vi "Camera.vi"(5 "Camera Notifiers":T2, 6 "Auto Settings?":bool, 7 "Refnums":T4, 8 "Error In":errorcluster, 9 "Set Camera ID":u32, 10 "Settings":T5={"Pixel clock"=20, "Frame rate"=30.0, "Exposure time"=33.21525, "Master Gain"=0, "Red Gain"=0, "Green Gain"=0, "Blue Gain"=0, "Auto Gain"=FALSE, "White-balance"=FALSE, "Color Correction"=FALSE} {"Blue Gain" min=0 max=100 step=1 scale=0.0..100.0; "Green Gain" min=0 max=100 step=1 scale=0.0..100.0; "Red Gain" min=0 max=100 step=1 scale=0.0..100.0; "Master Gain" min=0 max=100 step=1 scale=0.0..100.0; "Exposure time" min=0.271 max=424.65700000000004 step=0.271 scale=0.271..424.65700000000004 scale format="%#.3g"; "Frame rate" min=2.3503419747573275 max=2.3503419747573275 step=0.000271 scale=2.3503419747573275..2.5853761722330604 scale format="%^#_3g"; "Pixel clock" min=5 max=43 step=1 scale=5.0..43.0}, 11 "Function":T7=enum."Update Settings") -> (0 "Error Out":errorcluster, 2 "Image":T3(plugin-control), 3 "Image":T6)   [LabVIEW 2014]
uses:
  Camera Functions.ctl
  Camera Img Data.ctl
  Camera Settings.ctl
  Camera Refnums.ctl
  support/Instrument Status.ctl
  Camera Notifiers.ctl
  support/Instrument Status State.ctl
  <vilib>/vision/NI_Vision_Development_Module.lvlib
panel:
  out "Instrument Status":T1
  out "Camera Handle":u32=1
  # "LICENSED MATERIALS – PROPERTY OF IBM\nCopyright IBM Corp. 2016,\nALL RIGHTS RESERVED"
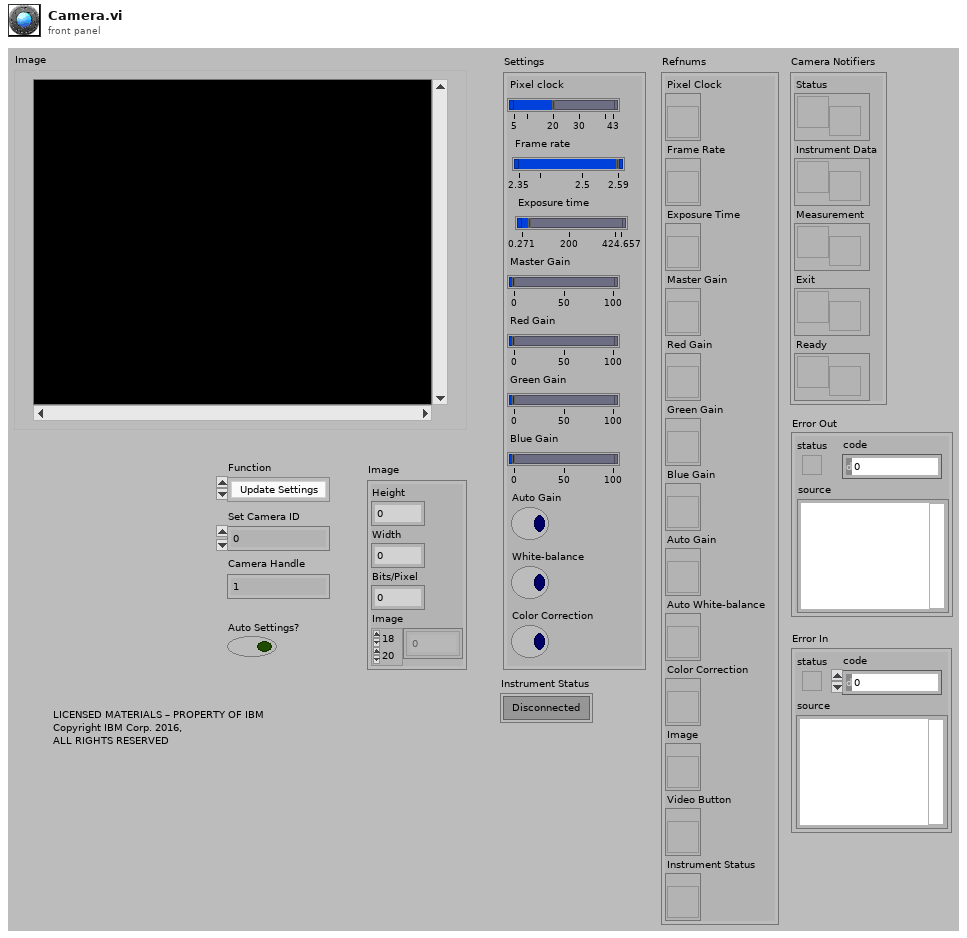
[diagram p1: front panel]
types:
  T1 = typedef "Instrument Status.ctl" = bool
  T2 = typedef "Camera Notifiers.ctl" = cluster{"Status":refnum<notifier>, "Instrument Data":refnum<notifier>, "Measurement":refnum<notifier>, "Exit":refnum<notifier>, "Ready":refnum<notifier>}
  T3 = typedef "IMAQ Image.ctl" = refnum<image>
  T4 = typedef "Camera Refnums.ctl" = cluster{"Pixel Clock":refnum<vi>, "Frame Rate":refnum<vi>, "Exposure Time":refnum<vi>, "Master Gain":refnum<vi>, "Red Gain":refnum<vi>, "Green Gain":refnum<vi>, "Blue Gain":refnum<vi>, "Auto Gain":refnum<vi>, "Auto White-balance":refnum<vi>, "Color Correction":refnum<vi>, "Image":refnum<vi>, "Video Button":refnum<vi>, "Instrument Status":refnum<vi>}
  T5 = typedef "Camera Settings.ctl" = cluster{"Pixel clock":i32, "Frame rate":dbl, "Exposure time":dbl, "Master Gain":i32, "Red Gain":i32, "Green Gain":i32, "Blue Gain":i32, "Auto Gain":bool, "White-balance":bool, "Color Correction":bool}
  T6 = typedef "Camera Img Data.ctl" = cluster{"Height":i32, "Width":i32, "Bits/Pixel":i32, "Image":u32[][]}
  T7 = typedef "Camera Functions.ctl" = enum16{"Connect", "Start Live", "Acquire", "Update Settings", "Update Settings2", "Stop Live", "Disconnect", "Update Refnums"}
  T8 = enum16{"All", "Limits", "Value", "User Enablement"}
  T9 = typedef "Instrument Status State.ctl" = enum16{"Unknown", "Idle", "Standby", "Configuring", "Measuring", "Moving", "Disconnected"}
  T10 = typedef "Image Type" = u32
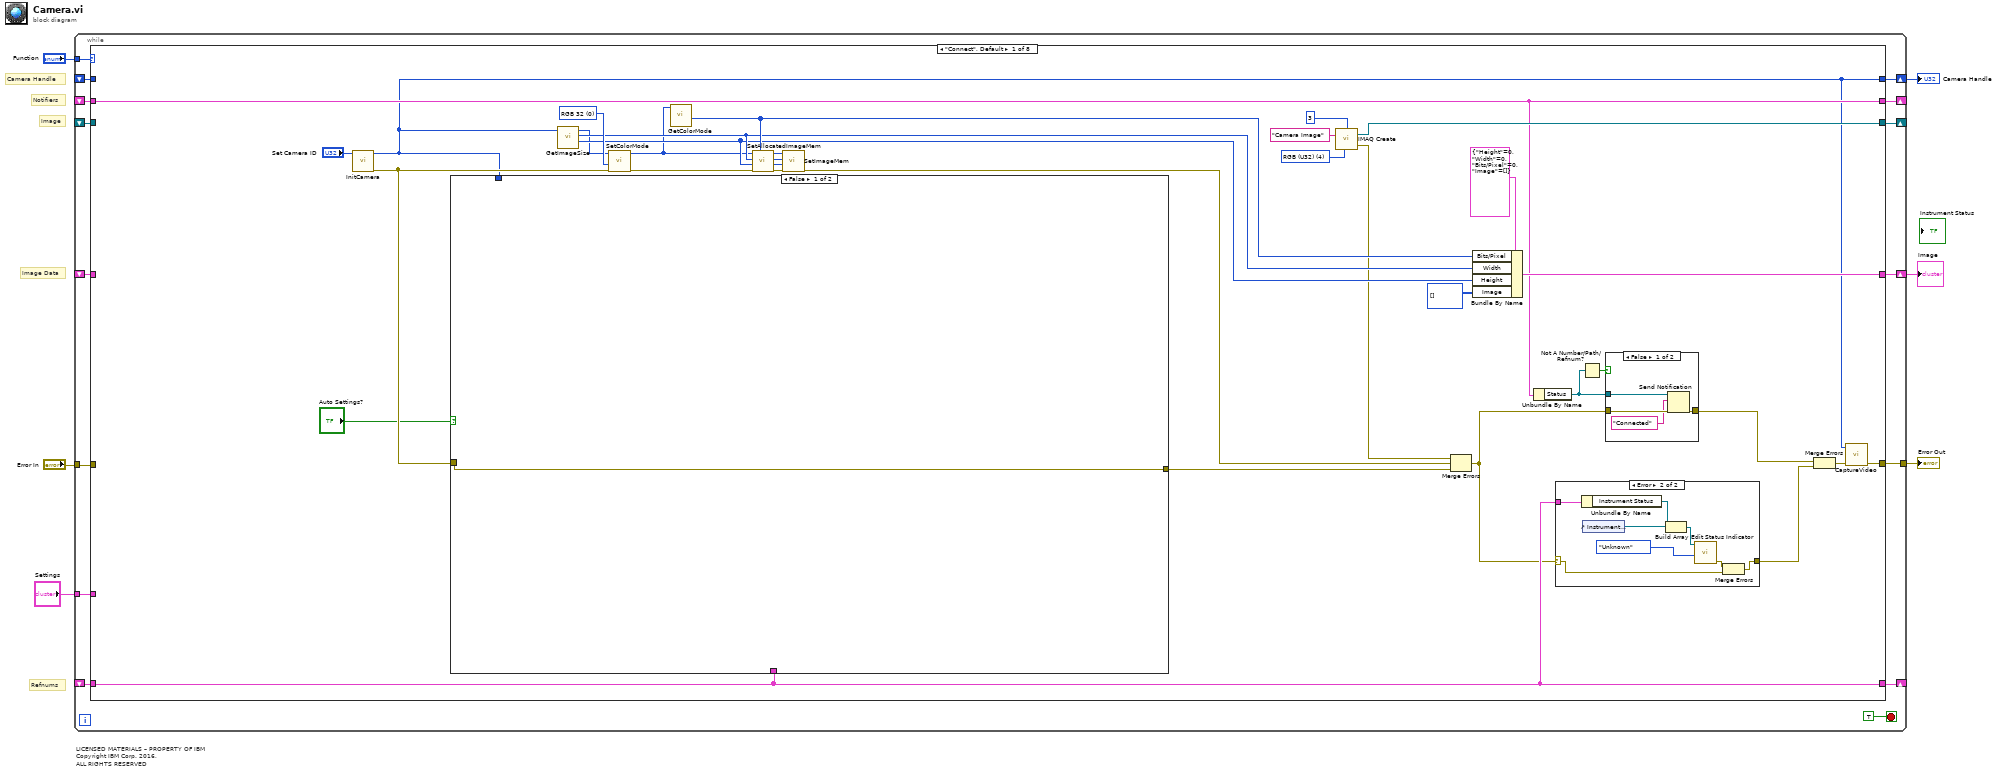
[diagram p0: block diagram]
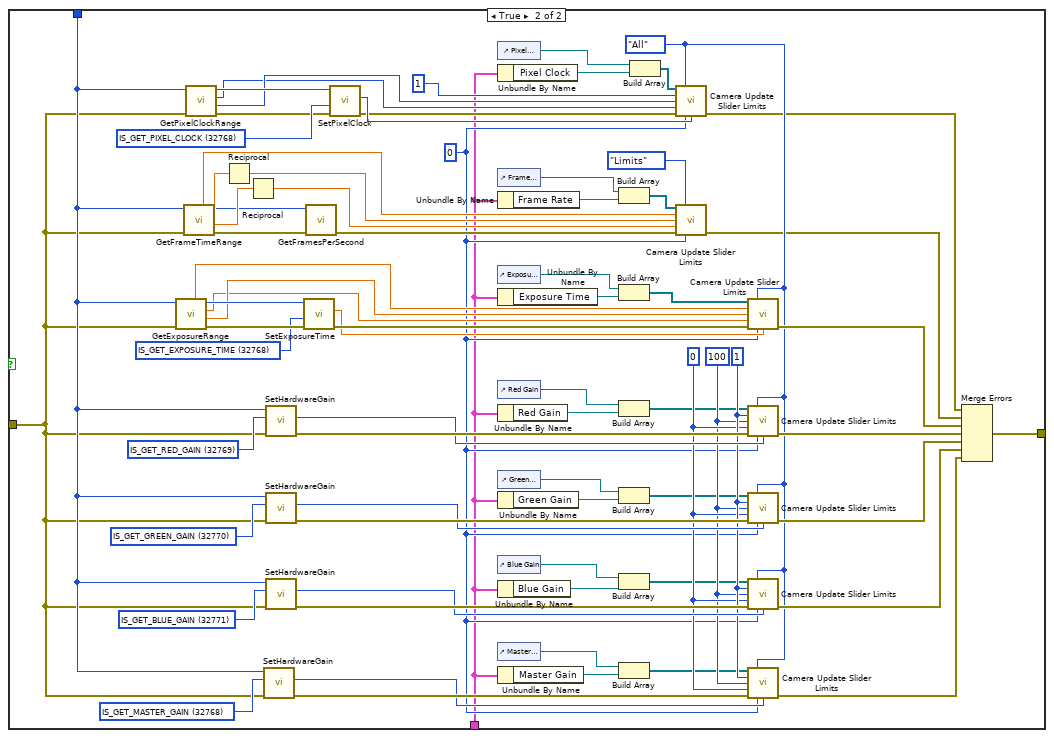
[diagram p2: hidden frame]
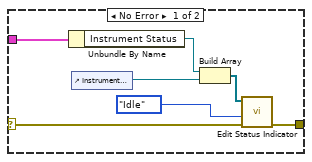
[diagram p3: hidden frame]
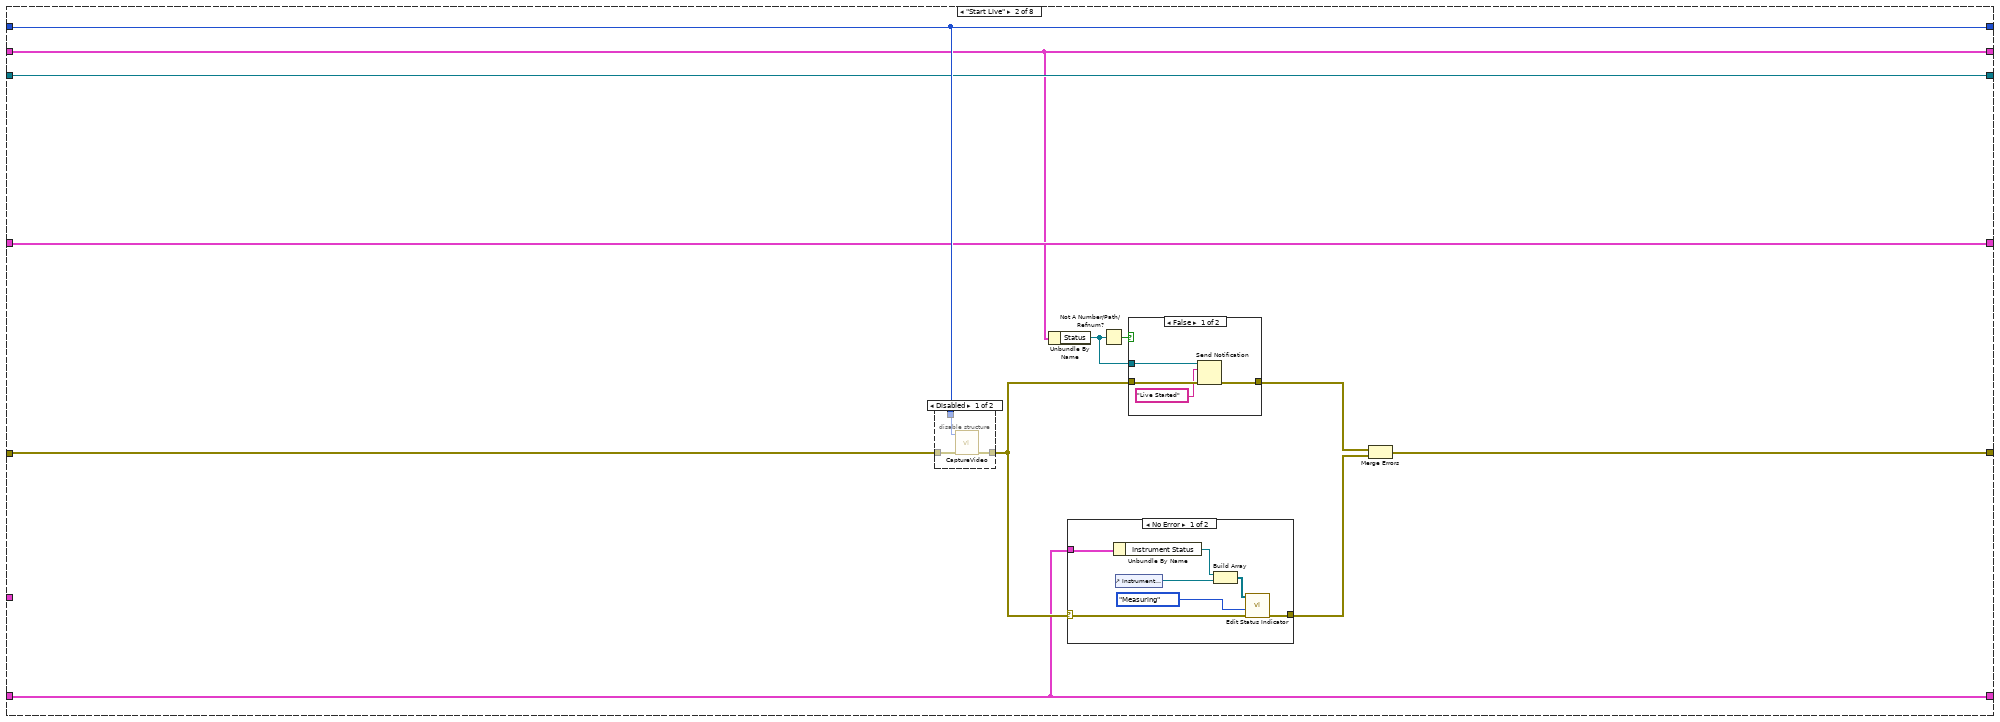
[diagram p5: hidden frame]
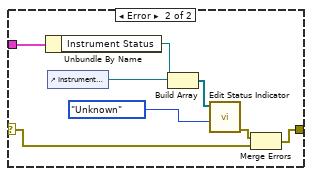
[diagram p7: hidden frame]
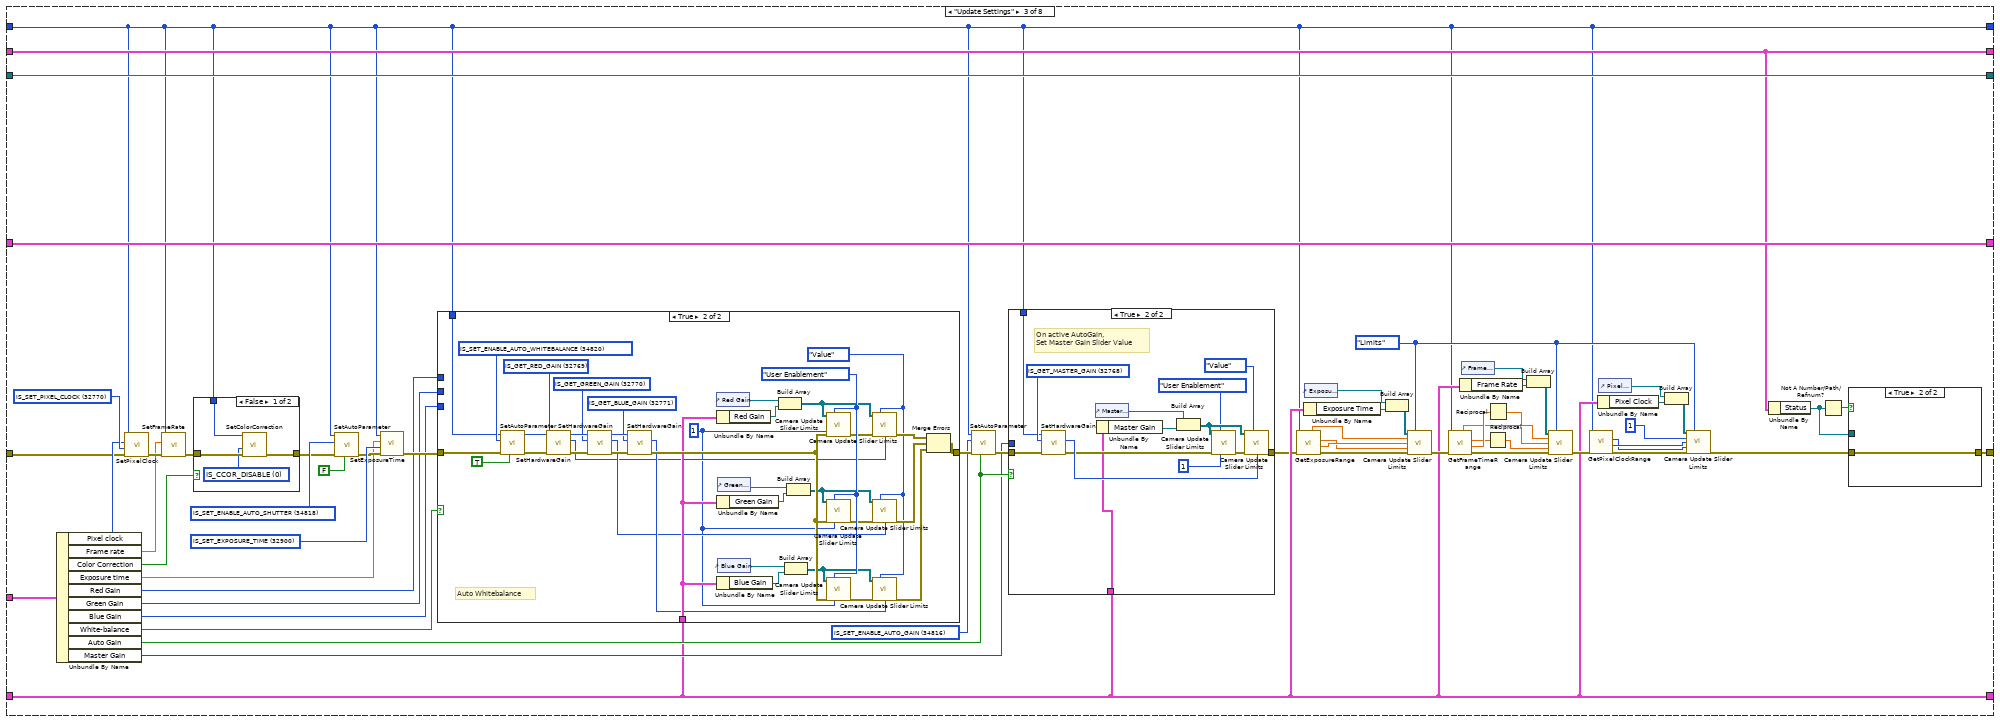
[diagram p9: hidden frame]
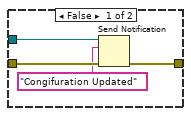
[diagram p10: hidden frame]
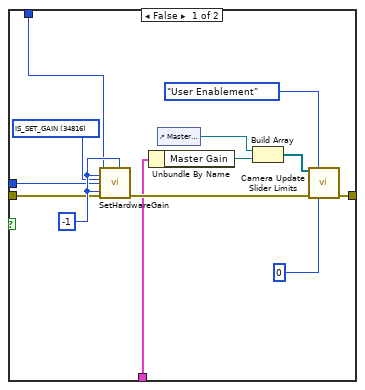
[diagram p11: hidden frame]
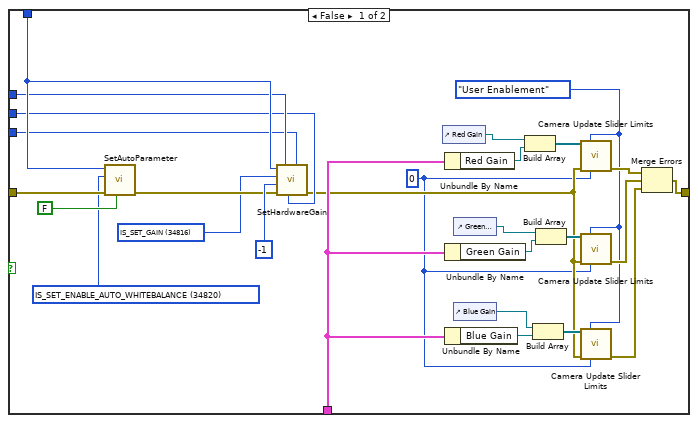
[diagram p12: hidden frame]
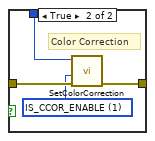
[diagram p13: hidden frame]
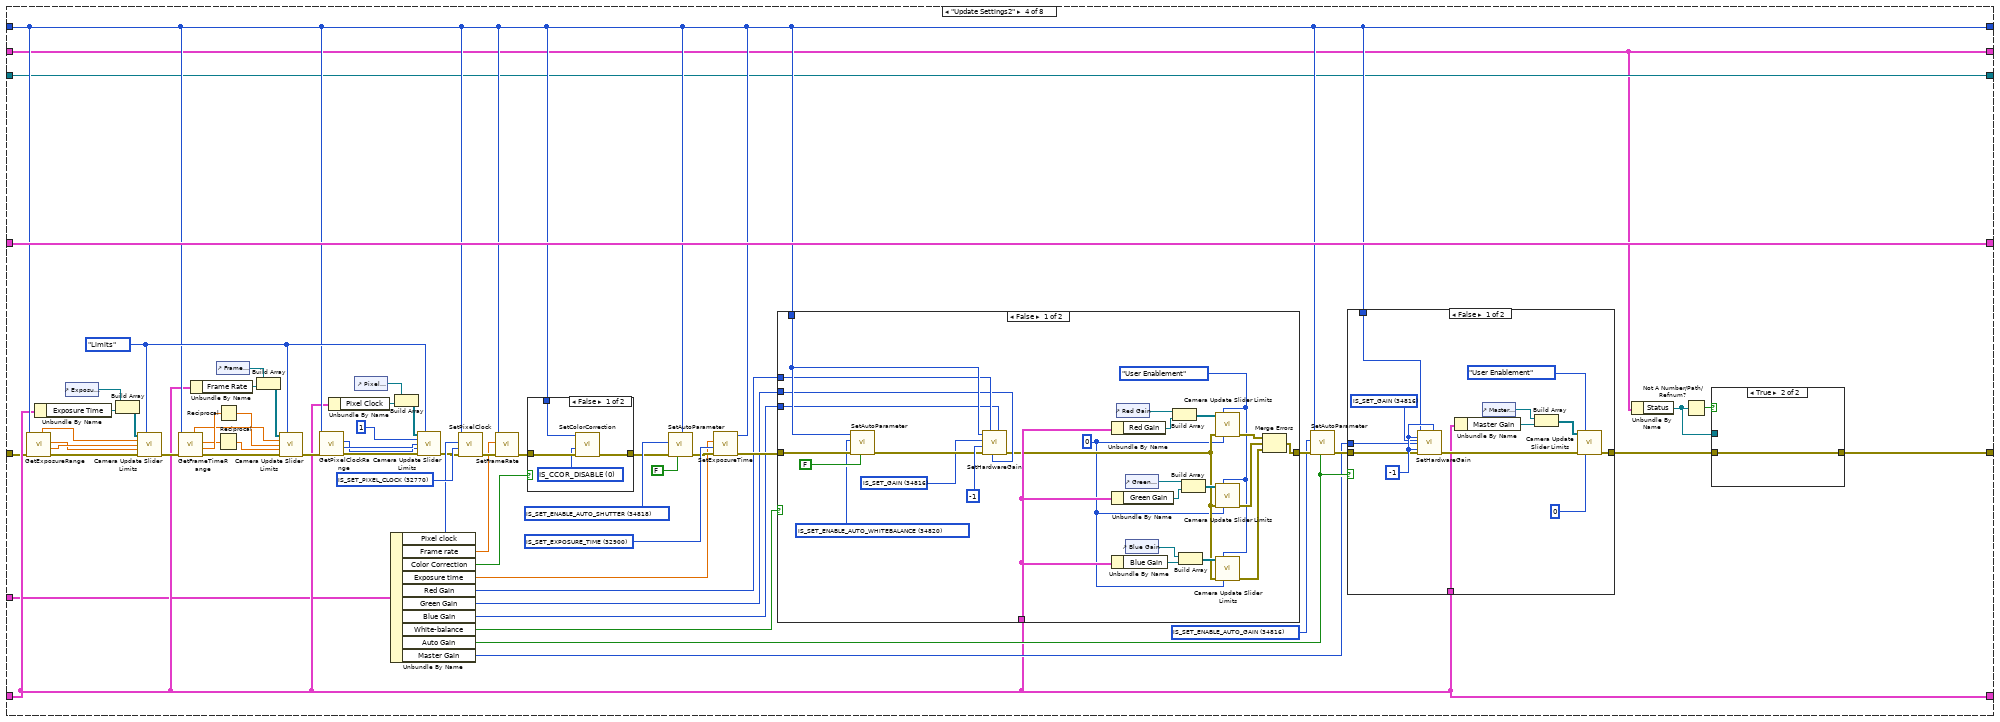
[diagram p14: hidden frame]
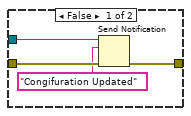
[diagram p15: hidden frame]
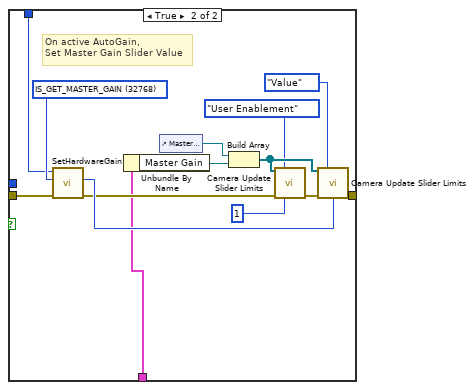
[diagram p16: hidden frame]
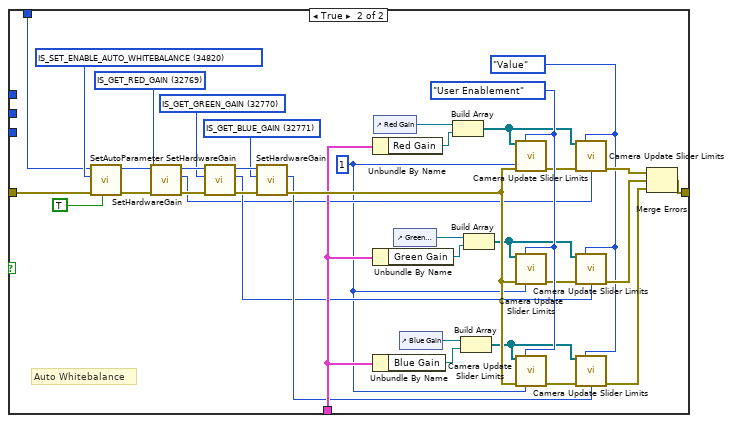
[diagram p17: hidden frame]
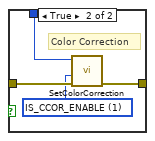
[diagram p18: hidden frame]
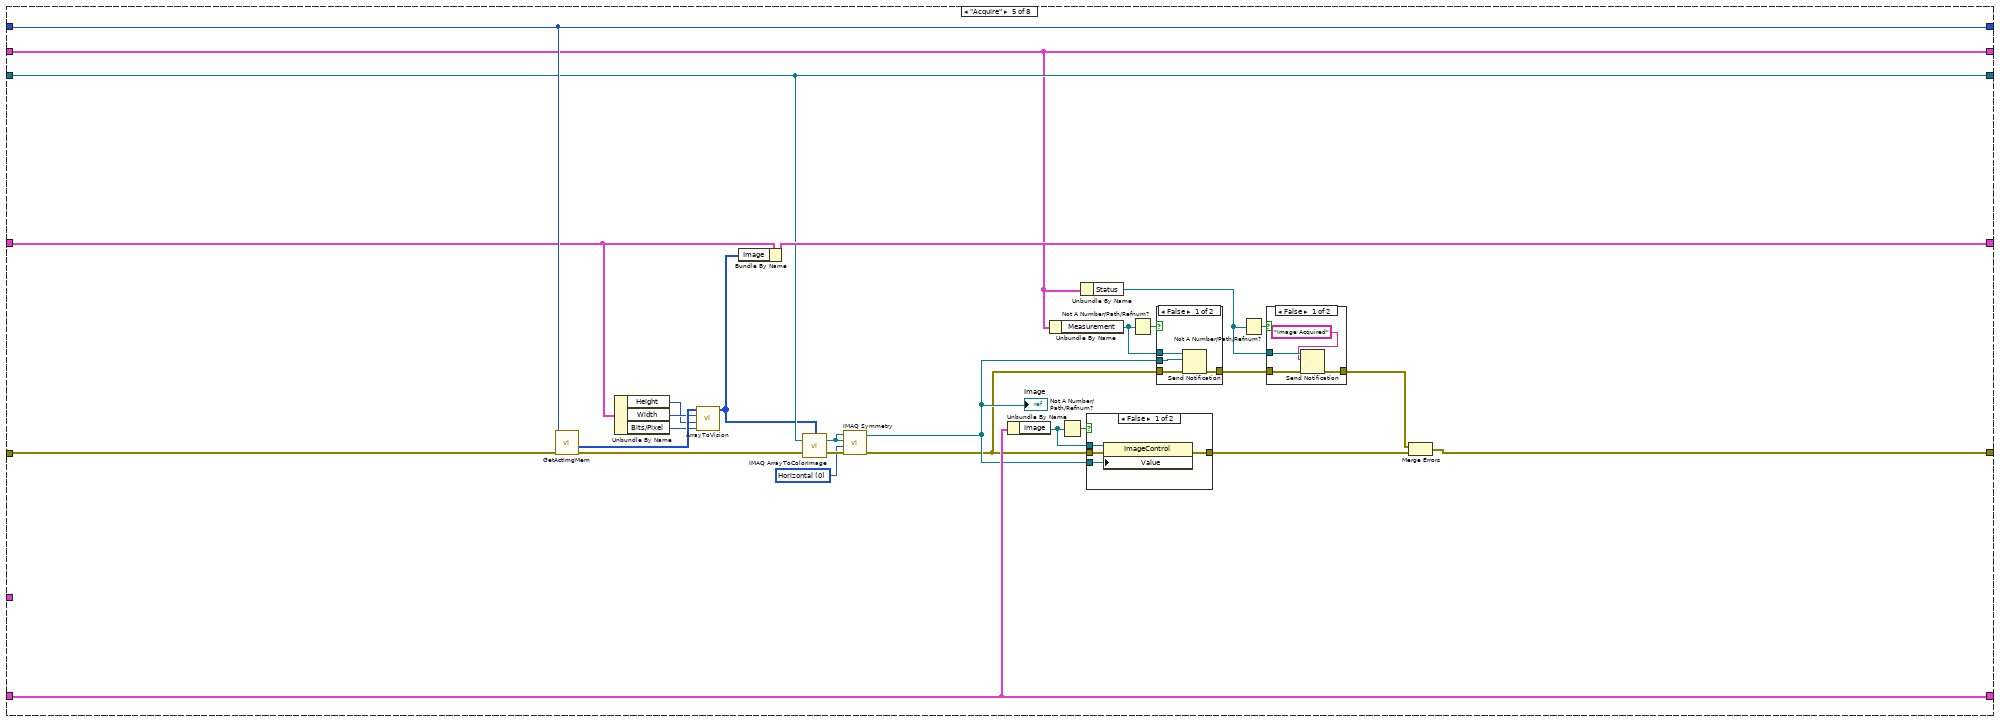
[diagram p19: hidden frame]
diagram:
  # "LICENSED MATERIALS – PROPERTY OF IBM\nCopyright IBM Corp. 2016,\nALL RIGHTS RESERVED"
  # "Notifiers"
  # "Image"
  # "Refnums"
  # "Image Data"
  # "Camera Handle"
  n1 = while {
    tunnel: [w21] -> w6
    tunnel: "Function" -> [w20]
    tunnel: "Error In" -> [w19]
    shift-right: [w17] -> w2
    shift-left: _ -> [w16]
    shift-right: [w12] -> w3
    shift-left: _ -> [w15]
    shift-right: [w14] -> _
    shift-left: _ -> [w13]
    shift-right: [w11] -> _
    shift-left: _ -> [w10]
    shift-right: [w8] -> _
    shift-left: _ -> [w9]
    tunnel: "Settings" -> [w7]
    stop <- TRUE stop-if-true
    n2 = case shown="\"Connect\", Default" w20 {
      tunnel: w19 -> [_ w161 w192 w351 w535 w574 w611 w635]
      tunnel: [w22 w154 w196 w354 w521 w565 w601 w635] -> w21
      tunnel: [w24 w162 w191 w359 w540 w558 w609 w640] -> w17
      tunnel: w16 -> [_ w162 w191 w359 w540 w558 w609 w640]
      tunnel: w15 -> [_ w160 w224 w388 w539 w572 w608 w639]
      tunnel: [w30 w151 w194 w352 w531 w561 w603 "Refnums"] -> w14
      tunnel: w13 -> [w30 w151 w194 w352 w531 w561 w603 _]
      tunnel: [w48 w160 w224 w388 w534 w572 w608 w639] -> w12
      tunnel: [w35 w159 w199 w358 w533 w571 w607 w638] -> w11
      tunnel: w10 -> [_ w159 w199 w358 w533 w571 w607 w638]
      tunnel: w9 -> [w31 w156 w195 w353 w523 w566 w604 _]
      tunnel: [w31 w156 w195 w353 w523 w566 w604 "Camera Notifiers"] -> w8
      tunnel: w7 -> [_ _ w193 w350 _ _ _ _]
      frame "Connect", Default {
        w37 = T10 4 items=["Grayscale (U8)", "Grayscale (I16)", "Grayscale (SGL)", "Complex (CSG)", "RGB (U32)", "HSL (U32)", "RGB (U64)", "Grayscale (U16)"] ("Image Type")
        w47 = 0 items=["RGB 32"=0, "RGB 24"=1, "Y8 Monochrom"=6] ("Mode")
        n3 = call <instrlib>:"InitCamera.vi"("Camera ID"="Set Camera ID") -> ("error out"=w40:errorcluster, "Camera Handle Out"=w24:u32)  [unwired: 9 out]
        n4 = case shown="False" "Auto Settings?" {
          tunnel: w24 -> [_ w66]
          tunnel: w40 -> [w56 w59]
          tunnel: w30 -> [_ w58]
          tunnel: [w56 w57] -> w27
          frame False {
          }
          frame True {
            w65 = T8."All" ("Edit?")
            w81 = 1 ("Maximum")
            w80 = 0 ("Minimum")
            w79 = 100 ("Maximum")
            w60 = u8 0
            w117 = 32768 items=["IS_GET_MASTER_GAIN"=32768, "IS_GET_RED_GAIN"=32769, "IS_GET_GREEN_GAIN"=32770, "IS_GET_BLUE_GAIN"=32771, "IS_GET_DEFAULT_MASTER"=32772, "IS_GET_DEFAULT_RED"=32773, "IS_GET_DEFAULT_GREEN"=32774, "IS_GET_DEFAULT_BLUE"=32775, "IS_SET_GAIN"=34816] ("Mode")
            w122 = u16 32768 items=["IS_SET_EXPOSURE_TIME"=32900, "IS_GET_EXPOSURE_TIME"=32768, "IS_GET_DEFAULT_EXPOSURE"=32769] ("Mode")
            w130 = 32771 items=["IS_GET_MASTER_GAIN"=32768, "IS_GET_RED_GAIN"=32769, "IS_GET_GREEN_GAIN"=32770, "IS_GET_BLUE_GAIN"=32771, "IS_GET_DEFAULT_MASTER"=32772, "IS_GET_DEFAULT_RED"=32773, "IS_GET_DEFAULT_GREEN"=32774, "IS_GET_DEFAULT_BLUE"=32775, "IS_SET_GAIN"=34816] ("Mode")
            w129 = 32770 items=["IS_GET_MASTER_GAIN"=32768, "IS_GET_RED_GAIN"=32769, "IS_GET_GREEN_GAIN"=32770, "IS_GET_BLUE_GAIN"=32771, "IS_GET_DEFAULT_MASTER"=32772, "IS_GET_DEFAULT_RED"=32773, "IS_GET_DEFAULT_GREEN"=32774, "IS_GET_DEFAULT_BLUE"=32775, "IS_SET_GAIN"=34816] ("Mode")
            w128 = 32769 items=["IS_GET_MASTER_GAIN"=32768, "IS_GET_RED_GAIN"=32769, "IS_GET_GREEN_GAIN"=32770, "IS_GET_BLUE_GAIN"=32771, "IS_GET_DEFAULT_MASTER"=32772, "IS_GET_DEFAULT_RED"=32773, "IS_GET_DEFAULT_GREEN"=32774, "IS_GET_DEFAULT_BLUE"=32775, "IS_SET_GAIN"=34816] ("Mode")
            w127 = 32768 items=["IS_GET_PIXEL_CLOCK"=32768, "IS_GET_DEFAULT_PCLK"=32769, "IS_SET_PIXEL_CLOCK"=32770] ("Mode")
            n5 = call <instrlib>:"GetExposureRange.vi"("error in"=w59, "Camera Handle In"=w66) -> ("error out"=w123:errorcluster, "max"=w105:dbl, "min"=w104:dbl, "Camera Handle Out"=w124:u32, "intervall"=w106:dbl)  [unwired: 5 out]
            n6 = call <instrlib>:"GetFrameTimeRange.vi"("error in"=w59, "Camera Handle In"=w66) -> ("error out"=w120:errorcluster, "max"=w125:dbl, "min"=w126:dbl, "Camera Handle Out"=w121:u32, "interval"=w116:dbl)  [unwired: 5 out]
            n7 = call <instrlib>:"GetPixelClockRange.vi"("error in"=w59, "Camera Handle In"=w66) -> ("error out"=w119:errorcluster, "Max"=w98:i32, "Min"=w97:i32, "Camera Handle Out"=w118:u32)  [unwired: 6 out]
            n8 = Reciprocal(x=w126) -> (1/x=w115:dbl)
            n9 = Reciprocal(x=w125) -> (1/x=w114:dbl)
            n10 = call <instrlib>:"SetHardwareGain.vi"("error in"=w59, "Mode"=w117, "Camera Handle In"=w66) -> ("error out"=w87:errorcluster, "Value"=w83:i32)  [unwired: 4 in, 3 out]
            n11 = call <instrlib>:"SetHardwareGain.vi"("error in"=w59, "Mode"=w128, "Camera Handle In"=w66) -> ("error out"=w93:errorcluster, "Value"=w82:i32)  [unwired: 4 in, 3 out]
            n12 = call <instrlib>:"SetHardwareGain.vi"("error in"=w59, "Mode"=w129, "Camera Handle In"=w66) -> ("error out"=w91:errorcluster, "Value"=w85:i32)  [unwired: 4 in, 3 out]
            n13 = call <instrlib>:"SetHardwareGain.vi"("error in"=w59, "Mode"=w130, "Camera Handle In"=w66) -> ("error out"=w89:errorcluster, "Value"=w84:i32)  [unwired: 4 in, 3 out]
            n14 = call <instrlib>:"SetExposureTime.vi"("error in"=w123, "Mode"=w122, "Camera Handle In"=w124) -> ("error out"=w110:errorcluster, "new exposure time"=w102:dbl)  [unwired: 1 in, 6 out]
            n15 = call <instrlib>:"GetFramesPerSecond.vi"("error in"=w120, "Camera Handle In"=w121) -> ("error out"=w111:errorcluster)  [unwired: 9 out]
            n16 = call <instrlib>:"SetPixelClock.vi"("error in"=w119, "Mode"=w127, "Camera Handle In"=w118) -> ("error out"=w94:errorcluster, "Value"=w99:i32)  [unwired: 1 in, 6 out]
            n17 = control-ref of="Pixel clock"() -> (w95:refnum<vi>)
            n18 = Unbundle By Name(w58) -> ("Pixel Clock"=w100:refnum<vi>)
            n19 = control-ref of="Frame rate"() -> (w112:refnum<vi>)
            n20 = Unbundle By Name(w58) -> ("Frame Rate"=w113:refnum<vi>)
            n21 = control-ref of="Exposure time"() -> (w108:refnum<vi>)
            n22 = Unbundle By Name(w58) -> ("Exposure Time"=w109:refnum<vi>)
            n23 = control-ref of="Red Gain"() -> (w73:refnum<vi>)
            n24 = Unbundle By Name(w58) -> ("Red Gain"=w78:refnum<vi>)
            n25 = control-ref of="Green Gain"() -> (w72:refnum<vi>)
            n26 = Unbundle By Name(w58) -> ("Green Gain"=w77:refnum<vi>)
            n27 = control-ref of="Blue Gain"() -> (w71:refnum<vi>)
            n28 = Unbundle By Name(w58) -> ("Blue Gain"=w76:refnum<vi>)
            n29 = control-ref of="Master Gain"() -> (w74:refnum<vi>)
            n30 = Unbundle By Name(w58) -> ("Master Gain"=w75:refnum<vi>)
            n31 = Build Array(w112, w113) -> (w64:refnum<vi>[])
            n32 = Build Array(w108, w109) -> (w107:refnum<vi>[])
            n33 = Build Array(w73, w78) -> (w70:refnum<vi>[])
            n34 = Build Array(w72, w77) -> (w69:refnum<vi>[])
            n35 = Build Array(w71, w76) -> (w68:refnum<vi>[])
            n36 = Build Array(w74, w75) -> (w67:refnum<vi>[])
            n37 = Build Array(w95, w100) -> (w101:refnum<vi>[])
            n38 = call "Camera Update Slider Limits.vi"("Refnums"=w101, "Edit?"=w65, "Data Entry Limits:Increment"=1 ("Value"), "Data Entry Limits:Maximum"=w98, "Data Entry Limits:Minimum"=w97, "error in (no error)"=w94, "Disabled"=w60, "Value"=w99) -> ("error out"=w63:errorcluster)  [unwired: 1 in, 6 out]
            n39 = call "Camera Update Slider Limits.vi"("Refnums"=w64, "Edit?"=T8."Limits", "Data Entry Limits:Increment"=w116, "Data Entry Limits:Maximum"=w115, "Data Entry Limits:Minimum"=w114, "error in (no error)"=w111, "Disabled"=w60) -> ("error out"=w61:errorcluster)  [unwired: 1 in, 7 out]
            n40 = call "Camera Update Slider Limits.vi"("Refnums"=w107, "Edit?"=w65, "Data Entry Limits:Increment"=w106, "Data Entry Limits:Maximum"=w105, "Data Entry Limits:Minimum"=w104, "error in (no error)"=w110, "Disabled"=w60, "Value"=w102) -> ("error out"=w103:errorcluster)  [unwired: 1 in, 6 out]
            n41 = call "Camera Update Slider Limits.vi"("Refnums"=w70, "Edit?"=w65, "Data Entry Limits:Increment"=w81, "Data Entry Limits:Maximum"=w79, "Data Entry Limits:Minimum"=w80, "error in (no error)"=w93, "Disabled"=w60, "Value"=w82) -> ("error out"=w92:errorcluster)  [unwired: 1 in, 6 out]
            n42 = call "Camera Update Slider Limits.vi"("Refnums"=w69, "Edit?"=w65, "Data Entry Limits:Increment"=w81, "Data Entry Limits:Maximum"=w79, "Data Entry Limits:Minimum"=w80, "error in (no error)"=w91, "Disabled"=w60, "Value"=w85) -> ("error out"=w90:errorcluster)  [unwired: 1 in, 6 out]
            n43 = call "Camera Update Slider Limits.vi"("Refnums"=w68, "Edit?"=w65, "Data Entry Limits:Increment"=w81, "Data Entry Limits:Maximum"=w79, "Data Entry Limits:Minimum"=w80, "error in (no error)"=w89, "Disabled"=w60, "Value"=w84) -> ("error out"=w88:errorcluster)  [unwired: 1 in, 6 out]
            n44 = call "Camera Update Slider Limits.vi"("Refnums"=w67, "Edit?"=w65, "Data Entry Limits:Increment"=w81, "Data Entry Limits:Maximum"=w79, "Data Entry Limits:Minimum"=w80, "error in (no error)"=w87, "Disabled"=w60, "Value"=w83) -> ("error out"=w86:errorcluster)  [unwired: 1 in, 6 out]
            n45 = Merge Errors(w63, w61, w103, w92, w90, w88, w86) -> (w57:errorcluster)
          }
        }
        n46 = call <instrlib>:"GetImageSize.vi"("Camera Handle In"=w24) -> ("Height"=w43:i32, "Width"=w44:i32, "Camera Handle Out"=w42:u32)  [unwired: 1 in, 7 out]
        n47 = call <instrlib>:"SetColorMode.vi"("error in"=w40, "Mode"=w47, "Camera Handle In"=w42) -> ("error out"=w46:errorcluster, "Camera Handle Out"=w41:u32)  [unwired: 7 out]
        n48 = call <instrlib>:"GetColorMode.vi"("Camera Handle In"=w41) -> ("Bits/Pixel"=w45:i32)  [unwired: 1 in, 9 out]
        n49 = call <instrlib>:"SetAllocatedImageMem.vi"("BitsPixel"=w45, "error in"=w46, "Height"=w43, "Width"=w44, "Camera Handle In"=w41) -> ("error out"=w52:errorcluster, "Image Memory Out"=w53:u8[], "Memory ID Out"=w54:i32, "Camera Handle Out"=w55:u32)  [unwired: 3 out]
        n50 = call <instrlib>:"SetImageMem.vi"("error in"=w52, "Image Memory In"=w53, "Memory ID In"=w54, "Camera Handle In"=w55) -> ("error out"=w26:errorcluster)  [unwired: 7 out]
        n51 = call "IMAQ Create"("Border Size"=3, "Image Name"="Camera Image", "Image Type"=w37) -> ("New Image"=w35:T3, "error out"=w36:errorcluster)  [unwired: 1 in, 1 out]
        n52 = Merge Errors(w36, w26, w27) -> (w29:errorcluster)
        n53 = Bundle By Name(cluster=T6 {"Height"=0, "Width"=0, "Bits/Pixel"=0, "Image"=[]} ("Image Data"), "Bits/Pixel"=w45, "Width"=w44, "Height"=w43, "Image"=u32[][] [] ("OutArray")) -> (w48:T6)
        n54 = Unbundle By Name(w31) -> ("Status"=w33:refnum<notifier>)
        n55 = case shown="Error" w29 {
          selector: w29 -> [w136 w141]
          tunnel: [w135 w140] -> w28
          tunnel: w30 -> [w132 w142]
          frame No Error {
            n56 = Unbundle By Name(w132) -> ("Instrument Status"=w133:refnum<vi>)
            n57 = control-ref of="Instrument Status"() -> (w131:refnum<vi>)
            n58 = Build Array(w133, w131) -> (w134:refnum<vi>[])
            n59 = call "Edit Status Indicator.vi"("error in (no error)"=w136, "State"=Instrument_Status_State."Idle", "Instrument Status Refnum"=w134) -> ("error out"=w135:errorcluster)  [unwired: 1 in, 7 out]
          }
          frame Error {
            n60 = Unbundle By Name(w142) -> ("Instrument Status"=w143:refnum<vi>)
            n61 = control-ref of="Instrument Status"() -> (w138:refnum<vi>)
            n62 = Build Array(w143, w138) -> (w144:refnum<vi>[])
            n63 = call "Edit Status Indicator.vi"("State"=Instrument_Status_State."Unknown", "Instrument Status Refnum"=w144) -> ("error out"=w139:errorcluster)  [unwired: 2 in, 7 out]
            n64 = Merge Errors(w139, w141) -> (w140:errorcluster)
          }
        }
        n65 = Not A Number/Path/Refnum?(number/path/refnum=w33) -> (NaN/Path/Refnum?=w34:bool)
        n66 = case shown="False" w34 {
          tunnel: w29 -> [w149 w150]
          tunnel: [w148 w150] -> w32
          tunnel: w33 -> [w147 _]
          frame False {
            n67 = Send Notification(notification="Connected", notifier=w147, error in (no error)=w149) -> (error out=w148:errorcluster)  [unwired: 1 out]
          }
          frame True {
          }
        }
        n68 = Merge Errors(w32, w28) -> (w23:errorcluster)
        n69 = call <instrlib>:"CaptureVideo.vi"("error in"=w23, "Camera Handle In"=w24) -> ("error out"=w22:errorcluster)  [unwired: 1 in, 8 out]
      }
      frame "Start Live" {
        n70 = disable-structure shown="Disabled" {
          disable-tunnel: w162 -> [w165 _]
          disable-tunnel: w161 -> [w164 _]
          disable-tunnel: [w163 _] -> w152
          frame Disabled {
            n71 = call <instrlib>:"CaptureVideo.vi"("error in"=w164, "Camera Handle In"=w165) -> ("error out"=w163:errorcluster)  [unwired: 1 in, 8 out]
          }
          frame Enabled {
          }
        }
        n72 = Unbundle By Name(w156) -> ("Status"=w157:refnum<notifier>)
        n73 = case shown="No Error" w152 {
          selector: w152 -> [w171 w176]
          tunnel: [w170 w175] -> w153
          tunnel: w151 -> [w167 w177]
          frame No Error {
            n74 = Unbundle By Name(w167) -> ("Instrument Status"=w168:refnum<vi>)
            n75 = control-ref of="Instrument Status"() -> (w166:refnum<vi>)
            n76 = Build Array(w168, w166) -> (w169:refnum<vi>[])
            n77 = call "Edit Status Indicator.vi"("error in (no error)"=w171, "State"=Instrument_Status_State."Measuring", "Instrument Status Refnum"=w169) -> ("error out"=w170:errorcluster)  [unwired: 1 in, 7 out]
          }
          frame Error {
            n78 = Unbundle By Name(w177) -> ("Instrument Status"=w178:refnum<vi>)
            n79 = control-ref of="Instrument Status"() -> (w173:refnum<vi>)
            n80 = Build Array(w178, w173) -> (w179:refnum<vi>[])
            n81 = call "Edit Status Indicator.vi"("State"=Instrument_Status_State."Unknown", "Instrument Status Refnum"=w179) -> ("error out"=w174:errorcluster)  [unwired: 2 in, 7 out]
            n82 = Merge Errors(w174, w176) -> (w175:errorcluster)
          }
        }
        n83 = Not A Number/Path/Refnum?(number/path/refnum=w157) -> (NaN/Path/Refnum?=w158:bool)
        n84 = case shown="False" w158 {
          tunnel: w152 -> [w184 w185]
          tunnel: [w183 w185] -> w155
          tunnel: w157 -> [w182 _]
          frame False {
            n85 = Send Notification(notification="Live Started", notifier=w182, error in (no error)=w184) -> (error out=w183:errorcluster)  [unwired: 1 out]
          }
          frame True {
          }
        }
        n86 = Merge Errors(w155, w153) -> (w154:errorcluster)
      }
      frame "Update Settings" {
        w200 = T8."Limits" ("Edit?")
        w242 = u16 32900 items=["IS_SET_EXPOSURE_TIME"=32900, "IS_GET_EXPOSURE_TIME"=32768, "IS_GET_DEFAULT_EXPOSURE"=32769] ("Mode")
        w238 = 34818 items=["IS_SET_ENABLE_AUTO_GAIN"=34816, "IS_GET_ENABLE_AUTO_GAIN"=34817, "IS_SET_ENABLE_AUTO_SHUTTER"=34818, "IS_GET_ENABLE_AUTO_SHUTTER"=34819, "IS_SET_ENABLE_AUTO_WHITEBALANCE"=34820, "IS_GET_ENABLE_AUTO_WHITEBALANCE"=34821, "IS_SET_ENABLE_AUTO_FRAMERATE"=34822, "IS_GET_ENABLE_AUTO_FRAMERATE"=34823, "IS_SET_AUTO_REFERENCE"=32768, "IS_GET_AUTO_REFERENCE"=32769, "IS_SET_AUTO_GAIN_MAX"=32770, "IS_GET_AUTO_GAIN_MAX"=32771, "IS_SET_AUTO_SHUTTER_MAX"=32772, "IS_GET_AUTO_SHUTTER_MAX"=32773, "IS_SET_AUTO_SPEED"=32774, "IS_GET_AUTO_SPEED"=32775, "IS_SET_AUTO_WB_OFFSET"=32776, "IS_GET_AUTO_WB_OFFSET"=32777, "IS_SET_AUTO_WB_GAIN_RANGE"=32778, "IS_GET_AUTO_WB_GAIN_RANGE"=32779, "IS_SET_AUTO_WB_SPEED"=32780, "IS_GET_SUTO_WB_SPEED"=32781, "IS_SET_AUTO_WB_ONCE"=32782, "IS_GET_AUTO_WB_ONCE"=32783] ("Param")
        w241 = 34816 items=["IS_SET_ENABLE_AUTO_GAIN"=34816, "IS_GET_ENABLE_AUTO_GAIN"=34817, "IS_SET_ENABLE_AUTO_SHUTTER"=34818, "IS_GET_ENABLE_AUTO_SHUTTER"=34819, "IS_SET_ENABLE_AUTO_WHITEBALANCE"=34820, "IS_GET_ENABLE_AUTO_WHITEBALANCE"=34821, "IS_SET_ENABLE_AUTO_FRAMERATE"=34822, "IS_GET_ENABLE_AUTO_FRAMERATE"=34823, "IS_SET_AUTO_REFERENCE"=32768, "IS_GET_AUTO_REFERENCE"=32769, "IS_SET_AUTO_GAIN_MAX"=32770, "IS_GET_AUTO_GAIN_MAX"=32771, "IS_SET_AUTO_SHUTTER_MAX"=32772, "IS_GET_AUTO_SHUTTER_MAX"=32773, "IS_SET_AUTO_SPEED"=32774, "IS_GET_AUTO_SPEED"=32775, "IS_SET_AUTO_WB_OFFSET"=32776, "IS_GET_AUTO_WB_OFFSET"=32777, "IS_SET_AUTO_WB_GAIN_RANGE"=32778, "IS_GET_AUTO_WB_GAIN_RANGE"=32779, "IS_SET_AUTO_WB_SPEED"=32780, "IS_GET_SUTO_WB_SPEED"=32781, "IS_SET_AUTO_WB_ONCE"=32782, "IS_GET_AUTO_WB_ONCE"=32783] ("Param")
        w243 = 32770 items=["IS_GET_PIXEL_CLOCK"=32768, "IS_GET_DEFAULT_PCLK"=32769, "IS_SET_PIXEL_CLOCK"=32770] ("Mode")
        n87 = Unbundle By Name(w193) -> ("Pixel clock"=w223:i32, "Frame rate"=w233:dbl, "Color Correction"=w230:bool, "Exposure time"=w228:dbl, "Red Gain"=w229:i32, "Green Gain"=w232:i32, "Blue Gain"=w231:i32, "White-balance"=w227:bool, "Auto Gain"=w226:bool, "Master Gain"=w225:i32)
        n88 = call <instrlib>:"SetPixelClock.vi"("error in"=w192, "Mode"=w243, "Pixel Clock"=w223, "Camera Handle In"=w191) -> ("error out"=w240:errorcluster)  [unwired: 7 out]
        n89 = call <instrlib>:"SetFrameRate.vi"("error in"=w240, "FPS"=w233, "Camera Handle In"=w191) -> ("error out"=w239:errorcluster)  [unwired: 8 out]
        n90 = case shown="False" w230 {
          tunnel: w239 -> [w345 w349]
          tunnel: [w344 w348] -> w236
          tunnel: w191 -> [w342 w346]
          frame False {
            w343 = 0 items=["IS_CCOR_DISABLE", "IS_CCOR_ENABLE"] ("Mode")
            n91 = call <instrlib>:"SetColorCorrection.vi"("error in"=w345, "Mode"=w343, "Camera Handle In"=w342) -> ("error out"=w344:errorcluster)  [unwired: 8 out]
          }
          frame True {
            w347 = 1 items=["IS_CCOR_DISABLE", "IS_CCOR_ENABLE"] ("Mode")
            # "Color Correction"
            n92 = call <instrlib>:"SetColorCorrection.vi"("error in"=w349, "Mode"=w347, "Camera Handle In"=w346) -> ("error out"=w348:errorcluster)  [unwired: 8 out]
          }
        }
        n93 = call <instrlib>:"SetAutoParameter.vi"("enable"=FALSE, "error in"=w236, "Param"=w238, "Camera Handle In"=w191) -> ("error out"=w235:errorcluster)  [unwired: 1 in, 6 out]
        n94 = call <instrlib>:"SetExposureTime.vi"("error in"=w235, "Mode"=w242, "Exposure Time"=w228, "Camera Handle In"=w191) -> ("error out"=w234:errorcluster)  [unwired: 7 out]
        n95 = case shown="True" w227 {
          tunnel: w234 -> [w302 w337]
          tunnel: [w286 w324] -> w245
          tunnel: w229 -> [w297 _]
          tunnel: w232 -> [w296 _]
          tunnel: w231 -> [w295 _]
          tunnel: w191 -> [w298 w329]
          tunnel: w194 -> [w294 w322]
          frame False {
            w282 = T8."User Enablement" ("Edit?")
            w299 = 34816 items=["IS_GET_MASTER_GAIN"=32768, "IS_GET_RED_GAIN"=32769, "IS_GET_GREEN_GAIN"=32770, "IS_GET_BLUE_GAIN"=32771, "IS_GET_DEFAULT_MASTER"=32772, "IS_GET_DEFAULT_RED"=32773, "IS_GET_DEFAULT_GREEN"=32774, "IS_GET_DEFAULT_BLUE"=32775, "IS_SET_GAIN"=34816] ("Mode")
            w300 = 34820 items=["IS_SET_ENABLE_AUTO_GAIN"=34816, "IS_GET_ENABLE_AUTO_GAIN"=34817, "IS_SET_ENABLE_AUTO_SHUTTER"=34818, "IS_GET_ENABLE_AUTO_SHUTTER"=34819, "IS_SET_ENABLE_AUTO_WHITEBALANCE"=34820, "IS_GET_ENABLE_AUTO_WHITEBALANCE"=34821, "IS_SET_ENABLE_AUTO_FRAMERATE"=34822, "IS_GET_ENABLE_AUTO_FRAMERATE"=34823, "IS_SET_AUTO_REFERENCE"=32768, "IS_GET_AUTO_REFERENCE"=32769, "IS_SET_AUTO_GAIN_MAX"=32770, "IS_GET_AUTO_GAIN_MAX"=32771, "IS_SET_AUTO_SHUTTER_MAX"=32772, "IS_GET_AUTO_SHUTTER_MAX"=32773, "IS_SET_AUTO_SPEED"=32774, "IS_GET_AUTO_SPEED"=32775, "IS_SET_AUTO_WB_OFFSET"=32776, "IS_GET_AUTO_WB_OFFSET"=32777, "IS_SET_AUTO_WB_GAIN_RANGE"=32778, "IS_GET_AUTO_WB_GAIN_RANGE"=32779, "IS_SET_AUTO_WB_SPEED"=32780, "IS_GET_SUTO_WB_SPEED"=32781, "IS_SET_AUTO_WB_ONCE"=32782, "IS_GET_AUTO_WB_ONCE"=32783] ("Param")
            w281 = u8 0
            n96 = call <instrlib>:"SetAutoParameter.vi"("enable"=FALSE, "error in"=w302, "Param"=w300, "Camera Handle In"=w298) -> ("error out"=w301:errorcluster)  [unwired: 1 in, 6 out]
            n97 = call <instrlib>:"SetHardwareGain.vi"("Blue"=w295, "Green"=w296, "Red"=w297, "error in"=w301, "Master Gain"=-1, "Mode"=w299, "Camera Handle In"=w298) -> ("error out"=w287:errorcluster)  [unwired: 4 out]
            n98 = control-ref of="Red Gain"() -> (w280:refnum<vi>)
            n99 = Unbundle By Name(w294) -> ("Red Gain"=w291:refnum<vi>)
            n100 = Unbundle By Name(w294) -> ("Green Gain"=w292:refnum<vi>)
            n101 = Unbundle By Name(w294) -> ("Blue Gain"=w293:refnum<vi>)
            n102 = control-ref of="Green Gain"() -> (w279:refnum<vi>)
            n103 = control-ref of="Blue Gain"() -> (w278:refnum<vi>)
            n104 = Build Array(w280, w291) -> (w290:refnum<vi>[])
            n105 = Build Array(w278, w293) -> (w288:refnum<vi>[])
            n106 = Build Array(w279, w292) -> (w289:refnum<vi>[])
            n107 = call "Camera Update Slider Limits.vi"("Refnums"=w290, "Edit?"=w282, "error in (no error)"=w287, "Disabled"=w281) -> ("error out"=w285:errorcluster)  [unwired: 4 in, 7 out]
            n108 = call "Camera Update Slider Limits.vi"("Refnums"=w289, "Edit?"=w282, "error in (no error)"=w287, "Disabled"=w281) -> ("error out"=w284:errorcluster)  [unwired: 4 in, 7 out]
            n109 = call "Camera Update Slider Limits.vi"("Refnums"=w288, "Edit?"=w282, "error in (no error)"=w287, "Disabled"=w281) -> ("error out"=w283:errorcluster)  [unwired: 4 in, 7 out]
            n110 = Merge Errors(w285, w284, w283) -> (w286:errorcluster)
          }
          frame True {
            w315 = T8."Value" ("Edit?")
            w325 = T8."User Enablement" ("Edit?")
            w311 = u8 1
            w330 = 32771 items=["IS_GET_MASTER_GAIN"=32768, "IS_GET_RED_GAIN"=32769, "IS_GET_GREEN_GAIN"=32770, "IS_GET_BLUE_GAIN"=32771, "IS_GET_DEFAULT_MASTER"=32772, "IS_GET_DEFAULT_RED"=32773, "IS_GET_DEFAULT_GREEN"=32774, "IS_GET_DEFAULT_BLUE"=32775, "IS_SET_GAIN"=34816] ("Mode")
            w331 = 32770 items=["IS_GET_MASTER_GAIN"=32768, "IS_GET_RED_GAIN"=32769, "IS_GET_GREEN_GAIN"=32770, "IS_GET_BLUE_GAIN"=32771, "IS_GET_DEFAULT_MASTER"=32772, "IS_GET_DEFAULT_RED"=32773, "IS_GET_DEFAULT_GREEN"=32774, "IS_GET_DEFAULT_BLUE"=32775, "IS_SET_GAIN"=34816] ("Mode")
            w332 = 32769 items=["IS_GET_MASTER_GAIN"=32768, "IS_GET_RED_GAIN"=32769, "IS_GET_GREEN_GAIN"=32770, "IS_GET_BLUE_GAIN"=32771, "IS_GET_DEFAULT_MASTER"=32772, "IS_GET_DEFAULT_RED"=32773, "IS_GET_DEFAULT_GREEN"=32774, "IS_GET_DEFAULT_BLUE"=32775, "IS_SET_GAIN"=34816] ("Mode")
            w333 = 34820 items=["IS_SET_ENABLE_AUTO_GAIN"=34816, "IS_GET_ENABLE_AUTO_GAIN"=34817, "IS_SET_ENABLE_AUTO_SHUTTER"=34818, "IS_GET_ENABLE_AUTO_SHUTTER"=34819, "IS_SET_ENABLE_AUTO_WHITEBALANCE"=34820, "IS_GET_ENABLE_AUTO_WHITEBALANCE"=34821, "IS_SET_ENABLE_AUTO_FRAMERATE"=34822, "IS_GET_ENABLE_AUTO_FRAMERATE"=34823, "IS_SET_AUTO_REFERENCE"=32768, "IS_GET_AUTO_REFERENCE"=32769, "IS_SET_AUTO_GAIN_MAX"=32770, "IS_GET_AUTO_GAIN_MAX"=32771, "IS_SET_AUTO_SHUTTER_MAX"=32772, "IS_GET_AUTO_SHUTTER_MAX"=32773, "IS_SET_AUTO_SPEED"=32774, "IS_GET_AUTO_SPEED"=32775, "IS_SET_AUTO_WB_OFFSET"=32776, "IS_GET_AUTO_WB_OFFSET"=32777, "IS_SET_AUTO_WB_GAIN_RANGE"=32778, "IS_GET_AUTO_WB_GAIN_RANGE"=32779, "IS_SET_AUTO_WB_SPEED"=32780, "IS_GET_SUTO_WB_SPEED"=32781, "IS_SET_AUTO_WB_ONCE"=32782, "IS_GET_AUTO_WB_ONCE"=32783] ("Param")
            # "Auto Whitebalance"
            n111 = call <instrlib>:"SetAutoParameter.vi"("enable"=TRUE, "error in"=w337, "Param"=w333, "Camera Handle In"=w329) -> ("error out"=w336:errorcluster, "Camera Handle Out"=w340:u32)  [unwired: 1 in, 5 out]
            n112 = call <instrlib>:"SetHardwareGain.vi"("error in"=w336, "Mode"=w332, "Camera Handle In"=w340) -> ("error out"=w335:errorcluster, "Value"=w312:i32, "Camera Handle Out"=w339:u32)  [unwired: 4 in, 2 out]
            n113 = call <instrlib>:"SetHardwareGain.vi"("error in"=w335, "Mode"=w331, "Camera Handle In"=w339) -> ("error out"=w334:errorcluster, "Value"=w313:i32, "Camera Handle Out"=w338:u32)  [unwired: 4 in, 2 out]
            n114 = call <instrlib>:"SetHardwareGain.vi"("error in"=w334, "Mode"=w330, "Camera Handle In"=w338) -> ("error out"=w323:errorcluster, "Value"=w314:i32)  [unwired: 4 in, 3 out]
            n115 = control-ref of="Red Gain"() -> (w307:refnum<vi>)
            n116 = Unbundle By Name(w322) -> ("Red Gain"=w326:refnum<vi>)
            n117 = Unbundle By Name(w322) -> ("Green Gain"=w327:refnum<vi>)
            n118 = Unbundle By Name(w322) -> ("Blue Gain"=w328:refnum<vi>)
            n119 = control-ref of="Green Gain"() -> (w306:refnum<vi>)
            n120 = control-ref of="Blue Gain"() -> (w305:refnum<vi>)
            n121 = Build Array(w307, w326) -> (w310:refnum<vi>[])
            n122 = Build Array(w305, w328) -> (w308:refnum<vi>[])
            n123 = Build Array(w306, w327) -> (w309:refnum<vi>[])
            n124 = call "Camera Update Slider Limits.vi"("Refnums"=w310, "Edit?"=w325, "error in (no error)"=w323, "Disabled"=w311) -> ("error out"=w321:errorcluster)  [unwired: 4 in, 7 out]
            n125 = call "Camera Update Slider Limits.vi"("Refnums"=w309, "Edit?"=w325, "error in (no error)"=w323, "Disabled"=w311) -> ("error out"=w320:errorcluster)  [unwired: 4 in, 7 out]
            n126 = call "Camera Update Slider Limits.vi"("Refnums"=w308, "Edit?"=w325, "error in (no error)"=w323, "Disabled"=w311) -> ("error out"=w319:errorcluster)  [unwired: 4 in, 7 out]
            n127 = call "Camera Update Slider Limits.vi"("Refnums"=w310, "Edit?"=w315, "error in (no error)"=w321, "Value"=w312) -> ("error out"=w318:errorcluster)  [unwired: 4 in, 7 out]
            n128 = call "Camera Update Slider Limits.vi"("Refnums"=w309, "Edit?"=w315, "error in (no error)"=w320, "Value"=w313) -> ("error out"=w317:errorcluster)  [unwired: 4 in, 7 out]
            n129 = call "Camera Update Slider Limits.vi"("Refnums"=w308, "Edit?"=w315, "error in (no error)"=w319, "Value"=w314) -> ("error out"=w316:errorcluster)  [unwired: 4 in, 7 out]
            n130 = Merge Errors(w318, w317, w316) -> (w324:errorcluster)
          }
        }
        n131 = call <instrlib>:"SetAutoParameter.vi"("enable"=w226, "error in"=w245, "Param"=w241, "Camera Handle In"=w191) -> ("error out"=w244:errorcluster)  [unwired: 1 in, 6 out]
        n132 = case shown="True" w226 {
          tunnel: w244 -> [w262 w277]
          tunnel: [w253 w266] -> w190
          tunnel: w225 -> [w259 _]
          tunnel: w191 -> [w260 w275]
          tunnel: w194 -> [w252 w265]
          frame False {
            w261 = 34816 items=["IS_GET_MASTER_GAIN"=32768, "IS_GET_RED_GAIN"=32769, "IS_GET_GREEN_GAIN"=32770, "IS_GET_BLUE_GAIN"=32771, "IS_GET_DEFAULT_MASTER"=32772, "IS_GET_DEFAULT_RED"=32773, "IS_GET_DEFAULT_GREEN"=32774, "IS_GET_DEFAULT_BLUE"=32775, "IS_SET_GAIN"=34816] ("Mode")
            w263 = -1
            n133 = call <instrlib>:"SetHardwareGain.vi"("Blue"=w263, "Green"=w263, "Red"=w263, "error in"=w262, "Master Gain"=w259, "Mode"=w261, "Camera Handle In"=w260) -> ("error out"=w254:errorcluster)  [unwired: 4 out]
            n134 = Unbundle By Name(w252) -> ("Master Gain"=w258:refnum<vi>)
            n135 = control-ref of="Master Gain"() -> (w251:refnum<vi>)
            n136 = Build Array(w251, w258) -> (w257:refnum<vi>[])
            n137 = call "Camera Update Slider Limits.vi"("Refnums"=w257, "Edit?"=T8."User Enablement", "error in (no error)"=w254, "Disabled"=u8 0) -> ("error out"=w253:errorcluster)  [unwired: 4 in, 7 out]
          }
          frame True {
            w276 = 32768 items=["IS_GET_MASTER_GAIN"=32768, "IS_GET_RED_GAIN"=32769, "IS_GET_GREEN_GAIN"=32770, "IS_GET_BLUE_GAIN"=32771, "IS_GET_DEFAULT_MASTER"=32772, "IS_GET_DEFAULT_RED"=32773, "IS_GET_DEFAULT_GREEN"=32774, "IS_GET_DEFAULT_BLUE"=32775, "IS_SET_GAIN"=34816] ("Mode")
            # "On active AutoGain,\nSet Master Gain Slider Value"
            n138 = call <instrlib>:"SetHardwareGain.vi"("error in"=w277, "Mode"=w276, "Camera Handle In"=w275) -> ("error out"=w267:errorcluster, "Value"=w268:i32)  [unwired: 4 in, 3 out]
            n139 = control-ref of="Master Gain"() -> (w264:refnum<vi>)
            n140 = Unbundle By Name(w265) -> ("Master Gain"=w273:refnum<vi>)
            n141 = Build Array(w264, w273) -> (w274:refnum<vi>[])
            n142 = call "Camera Update Slider Limits.vi"("Refnums"=w274, "Edit?"=T8."User Enablement", "error in (no error)"=w267, "Disabled"=u8 1) -> ("error out"=w270:errorcluster)  [unwired: 4 in, 7 out]
            n143 = call "Camera Update Slider Limits.vi"("Refnums"=w274, "Edit?"=T8."Value", "error in (no error)"=w270, "Value"=w268) -> ("error out"=w266:errorcluster)  [unwired: 4 in, 7 out]
          }
        }
        n144 = call <instrlib>:"GetExposureRange.vi"("error in"=w190, "Camera Handle In"=w191) -> ("error out"=w215:errorcluster, "max"=w219:dbl, "min"=w218:dbl, "intervall"=w220:dbl)  [unwired: 6 out]
        n145 = Unbundle By Name(w194) -> ("Exposure Time"=w217:refnum<vi>)
        n146 = control-ref of="Exposure time"() -> (w188:refnum<vi>)
        n147 = Build Array(w188, w217) -> (w216:refnum<vi>[])
        n148 = call "Camera Update Slider Limits.vi"("Refnums"=w216, "Edit?"=w200, "Data Entry Limits:Increment"=w220, "Data Entry Limits:Maximum"=w219, "Data Entry Limits:Minimum"=w218, "error in (no error)"=w215) -> ("error out"=w209:errorcluster)  [unwired: 2 in, 7 out]
        n149 = call <instrlib>:"GetFrameTimeRange.vi"("error in"=w209, "Camera Handle In"=w191) -> ("error out"=w214:errorcluster, "max"=w222:dbl, "min"=w221:dbl, "interval"=w213:dbl)  [unwired: 6 out]
        n150 = Unbundle By Name(w194) -> ("Frame Rate"=w210:refnum<vi>)
        n151 = control-ref of="Frame rate"() -> (w187:refnum<vi>)
        n152 = Reciprocal(x=w221) -> (1/x=w211:dbl)
        n153 = Reciprocal(x=w222) -> (1/x=w212:dbl)
        n154 = Build Array(w187, w210) -> (w207:refnum<vi>[])
        n155 = call "Camera Update Slider Limits.vi"("Refnums"=w207, "Edit?"=w200, "Data Entry Limits:Increment"=w213, "Data Entry Limits:Maximum"=w212, "Data Entry Limits:Minimum"=w211, "error in (no error)"=w214) -> ("error out"=w208:errorcluster)  [unwired: 2 in, 7 out]
        n156 = call <instrlib>:"GetPixelClockRange.vi"("error in"=w208, "Camera Handle In"=w191) -> ("error out"=w206:errorcluster, "Max"=w205:i32, "Min"=w204:i32)  [unwired: 7 out]
        n157 = Unbundle By Name(w194) -> ("Pixel Clock"=w202:refnum<vi>)
        n158 = control-ref of="Pixel clock"() -> (w186:refnum<vi>)
        n159 = Build Array(w186, w202) -> (w201:refnum<vi>[])
        n160 = call "Camera Update Slider Limits.vi"("Refnums"=w201, "Edit?"=w200, "Data Entry Limits:Increment"=1, "Data Entry Limits:Maximum"=w205, "Data Entry Limits:Minimum"=w204, "error in (no error)"=w206) -> ("error out"=w189:errorcluster)  [unwired: 2 in, 7 out]
        n161 = Unbundle By Name(w195) -> ("Status"=w197:refnum<notifier>)
        n162 = Not A Number/Path/Refnum?(number/path/refnum=w197) -> (NaN/Path/Refnum?=w198:bool)
        n163 = case shown="True" w198 {
          tunnel: w189 -> [w249 w250]
          tunnel: [w248 w250] -> w196
          tunnel: w197 -> [w247 _]
          frame False {
            n164 = Send Notification(notification="Congifuration Updated", notifier=w247, error in (no error)=w249) -> (error out=w248:errorcluster)  [unwired: 1 out]
          }
          frame True {
          }
        }
      }
      frame "Update Settings2" {
        w364 = T8."Limits" ("Edit?")
        w406 = u16 32900 items=["IS_SET_EXPOSURE_TIME"=32900, "IS_GET_EXPOSURE_TIME"=32768, "IS_GET_DEFAULT_EXPOSURE"=32769] ("Mode")
        w402 = 34818 items=["IS_SET_ENABLE_AUTO_GAIN"=34816, "IS_GET_ENABLE_AUTO_GAIN"=34817, "IS_SET_ENABLE_AUTO_SHUTTER"=34818, "IS_GET_ENABLE_AUTO_SHUTTER"=34819, "IS_SET_ENABLE_AUTO_WHITEBALANCE"=34820, "IS_GET_ENABLE_AUTO_WHITEBALANCE"=34821, "IS_SET_ENABLE_AUTO_FRAMERATE"=34822, "IS_GET_ENABLE_AUTO_FRAMERATE"=34823, "IS_SET_AUTO_REFERENCE"=32768, "IS_GET_AUTO_REFERENCE"=32769, "IS_SET_AUTO_GAIN_MAX"=32770, "IS_GET_AUTO_GAIN_MAX"=32771, "IS_SET_AUTO_SHUTTER_MAX"=32772, "IS_GET_AUTO_SHUTTER_MAX"=32773, "IS_SET_AUTO_SPEED"=32774, "IS_GET_AUTO_SPEED"=32775, "IS_SET_AUTO_WB_OFFSET"=32776, "IS_GET_AUTO_WB_OFFSET"=32777, "IS_SET_AUTO_WB_GAIN_RANGE"=32778, "IS_GET_AUTO_WB_GAIN_RANGE"=32779, "IS_SET_AUTO_WB_SPEED"=32780, "IS_GET_SUTO_WB_SPEED"=32781, "IS_SET_AUTO_WB_ONCE"=32782, "IS_GET_AUTO_WB_ONCE"=32783] ("Param")
        w405 = 34816 items=["IS_SET_ENABLE_AUTO_GAIN"=34816, "IS_GET_ENABLE_AUTO_GAIN"=34817, "IS_SET_ENABLE_AUTO_SHUTTER"=34818, "IS_GET_ENABLE_AUTO_SHUTTER"=34819, "IS_SET_ENABLE_AUTO_WHITEBALANCE"=34820, "IS_GET_ENABLE_AUTO_WHITEBALANCE"=34821, "IS_SET_ENABLE_AUTO_FRAMERATE"=34822, "IS_GET_ENABLE_AUTO_FRAMERATE"=34823, "IS_SET_AUTO_REFERENCE"=32768, "IS_GET_AUTO_REFERENCE"=32769, "IS_SET_AUTO_GAIN_MAX"=32770, "IS_GET_AUTO_GAIN_MAX"=32771, "IS_SET_AUTO_SHUTTER_MAX"=32772, "IS_GET_AUTO_SHUTTER_MAX"=32773, "IS_SET_AUTO_SPEED"=32774, "IS_GET_AUTO_SPEED"=32775, "IS_SET_AUTO_WB_OFFSET"=32776, "IS_GET_AUTO_WB_OFFSET"=32777, "IS_SET_AUTO_WB_GAIN_RANGE"=32778, "IS_GET_AUTO_WB_GAIN_RANGE"=32779, "IS_SET_AUTO_WB_SPEED"=32780, "IS_GET_SUTO_WB_SPEED"=32781, "IS_SET_AUTO_WB_ONCE"=32782, "IS_GET_AUTO_WB_ONCE"=32783] ("Param")
        w407 = 32770 items=["IS_GET_PIXEL_CLOCK"=32768, "IS_GET_DEFAULT_PCLK"=32769, "IS_SET_PIXEL_CLOCK"=32770] ("Mode")
        n165 = call <instrlib>:"GetExposureRange.vi"("error in"=w351, "Camera Handle In"=w359) -> ("error out"=w379:errorcluster, "max"=w383:dbl, "min"=w382:dbl, "intervall"=w384:dbl)  [unwired: 6 out]
        n166 = Unbundle By Name(w352) -> ("Exposure Time"=w381:refnum<vi>)
        n167 = control-ref of="Exposure time"() -> (w360:refnum<vi>)
        n168 = Build Array(w360, w381) -> (w380:refnum<vi>[])
        n169 = call "Camera Update Slider Limits.vi"("Refnums"=w380, "Edit?"=w364, "Data Entry Limits:Increment"=w384, "Data Entry Limits:Maximum"=w383, "Data Entry Limits:Minimum"=w382, "error in (no error)"=w379) -> ("error out"=w373:errorcluster)  [unwired: 2 in, 7 out]
        n170 = call <instrlib>:"GetFrameTimeRange.vi"("error in"=w373, "Camera Handle In"=w359) -> ("error out"=w378:errorcluster, "max"=w386:dbl, "min"=w385:dbl, "interval"=w377:dbl)  [unwired: 6 out]
        n171 = Unbundle By Name(w352) -> ("Frame Rate"=w374:refnum<vi>)
        n172 = Reciprocal(x=w385) -> (1/x=w375:dbl)
        n173 = control-ref of="Frame rate"() -> (w361:refnum<vi>)
        n174 = Reciprocal(x=w386) -> (1/x=w376:dbl)
        n175 = Build Array(w361, w374) -> (w371:refnum<vi>[])
        n176 = call "Camera Update Slider Limits.vi"("Refnums"=w371, "Edit?"=w364, "Data Entry Limits:Increment"=w377, "Data Entry Limits:Maximum"=w376, "Data Entry Limits:Minimum"=w375, "error in (no error)"=w378) -> ("error out"=w372:errorcluster)  [unwired: 2 in, 7 out]
        n177 = call <instrlib>:"GetPixelClockRange.vi"("error in"=w372, "Camera Handle In"=w359) -> ("error out"=w370:errorcluster, "Max"=w369:i32, "Min"=w368:i32)  [unwired: 7 out]
        n178 = Unbundle By Name(w352) -> ("Pixel Clock"=w366:refnum<vi>)
        n179 = control-ref of="Pixel clock"() -> (w362:refnum<vi>)
        n180 = Unbundle By Name(w350) -> ("Pixel clock"=w387:i32, "Frame rate"=w397:dbl, "Color Correction"=w394:bool, "Exposure time"=w392:dbl, "Red Gain"=w393:i32, "Green Gain"=w396:i32, "Blue Gain"=w395:i32, "White-balance"=w391:bool, "Auto Gain"=w390:bool, "Master Gain"=w389:i32)
        n181 = Build Array(w362, w366) -> (w365:refnum<vi>[])
        n182 = call "Camera Update Slider Limits.vi"("Refnums"=w365, "Edit?"=w364, "Data Entry Limits:Increment"=1, "Data Entry Limits:Maximum"=w369, "Data Entry Limits:Minimum"=w368, "error in (no error)"=w370) -> ("error out"=w363:errorcluster)  [unwired: 2 in, 7 out]
        n183 = call <instrlib>:"SetPixelClock.vi"("error in"=w363, "Mode"=w407, "Pixel Clock"=w387, "Camera Handle In"=w359) -> ("error out"=w404:errorcluster)  [unwired: 7 out]
        n184 = call <instrlib>:"SetFrameRate.vi"("error in"=w404, "FPS"=w397, "Camera Handle In"=w359) -> ("error out"=w403:errorcluster)  [unwired: 8 out]
        n185 = case shown="False" w394 {
          tunnel: w403 -> [w509 w513]
          tunnel: [w508 w512] -> w400
          tunnel: w359 -> [w506 w510]
          frame False {
            w507 = 0 items=["IS_CCOR_DISABLE", "IS_CCOR_ENABLE"] ("Mode")
            n186 = call <instrlib>:"SetColorCorrection.vi"("error in"=w509, "Mode"=w507, "Camera Handle In"=w506) -> ("error out"=w508:errorcluster)  [unwired: 8 out]
          }
          frame True {
            w511 = 1 items=["IS_CCOR_DISABLE", "IS_CCOR_ENABLE"] ("Mode")
            # "Color Correction"
            n187 = call <instrlib>:"SetColorCorrection.vi"("error in"=w513, "Mode"=w511, "Camera Handle In"=w510) -> ("error out"=w512:errorcluster)  [unwired: 8 out]
          }
        }
        n188 = call <instrlib>:"SetAutoParameter.vi"("enable"=FALSE, "error in"=w400, "Param"=w402, "Camera Handle In"=w359) -> ("error out"=w399:errorcluster)  [unwired: 1 in, 6 out]
        n189 = call <instrlib>:"SetExposureTime.vi"("error in"=w399, "Mode"=w406, "Exposure Time"=w392, "Camera Handle In"=w359) -> ("error out"=w398:errorcluster)  [unwired: 7 out]
        n190 = case shown="False" w391 {
          tunnel: w398 -> [w466 w501]
          tunnel: [w450 w488] -> w409
          tunnel: w393 -> [w461 _]
          tunnel: w396 -> [w460 _]
          tunnel: w395 -> [w459 _]
          tunnel: w359 -> [w462 w493]
          tunnel: w352 -> [w458 w486]
          frame False {
            w446 = T8."User Enablement" ("Edit?")
            w463 = 34816 items=["IS_GET_MASTER_GAIN"=32768, "IS_GET_RED_GAIN"=32769, "IS_GET_GREEN_GAIN"=32770, "IS_GET_BLUE_GAIN"=32771, "IS_GET_DEFAULT_MASTER"=32772, "IS_GET_DEFAULT_RED"=32773, "IS_GET_DEFAULT_GREEN"=32774, "IS_GET_DEFAULT_BLUE"=32775, "IS_SET_GAIN"=34816] ("Mode")
            w464 = 34820 items=["IS_SET_ENABLE_AUTO_GAIN"=34816, "IS_GET_ENABLE_AUTO_GAIN"=34817, "IS_SET_ENABLE_AUTO_SHUTTER"=34818, "IS_GET_ENABLE_AUTO_SHUTTER"=34819, "IS_SET_ENABLE_AUTO_WHITEBALANCE"=34820, "IS_GET_ENABLE_AUTO_WHITEBALANCE"=34821, "IS_SET_ENABLE_AUTO_FRAMERATE"=34822, "IS_GET_ENABLE_AUTO_FRAMERATE"=34823, "IS_SET_AUTO_REFERENCE"=32768, "IS_GET_AUTO_REFERENCE"=32769, "IS_SET_AUTO_GAIN_MAX"=32770, "IS_GET_AUTO_GAIN_MAX"=32771, "IS_SET_AUTO_SHUTTER_MAX"=32772, "IS_GET_AUTO_SHUTTER_MAX"=32773, "IS_SET_AUTO_SPEED"=32774, "IS_GET_AUTO_SPEED"=32775, "IS_SET_AUTO_WB_OFFSET"=32776, "IS_GET_AUTO_WB_OFFSET"=32777, "IS_SET_AUTO_WB_GAIN_RANGE"=32778, "IS_GET_AUTO_WB_GAIN_RANGE"=32779, "IS_SET_AUTO_WB_SPEED"=32780, "IS_GET_SUTO_WB_SPEED"=32781, "IS_SET_AUTO_WB_ONCE"=32782, "IS_GET_AUTO_WB_ONCE"=32783] ("Param")
            w445 = u8 0
            n191 = call <instrlib>:"SetAutoParameter.vi"("enable"=FALSE, "error in"=w466, "Param"=w464, "Camera Handle In"=w462) -> ("error out"=w465:errorcluster)  [unwired: 1 in, 6 out]
            n192 = call <instrlib>:"SetHardwareGain.vi"("Blue"=w459, "Green"=w460, "Red"=w461, "error in"=w465, "Master Gain"=-1, "Mode"=w463, "Camera Handle In"=w462) -> ("error out"=w451:errorcluster)  [unwired: 4 out]
            n193 = Unbundle By Name(w458) -> ("Red Gain"=w455:refnum<vi>)
            n194 = Unbundle By Name(w458) -> ("Green Gain"=w456:refnum<vi>)
            n195 = Unbundle By Name(w458) -> ("Blue Gain"=w457:refnum<vi>)
            n196 = control-ref of="Red Gain"() -> (w444:refnum<vi>)
            n197 = control-ref of="Green Gain"() -> (w443:refnum<vi>)
            n198 = control-ref of="Blue Gain"() -> (w442:refnum<vi>)
            n199 = Build Array(w444, w455) -> (w454:refnum<vi>[])
            n200 = Build Array(w442, w457) -> (w452:refnum<vi>[])
            n201 = Build Array(w443, w456) -> (w453:refnum<vi>[])
            n202 = call "Camera Update Slider Limits.vi"("Refnums"=w454, "Edit?"=w446, "error in (no error)"=w451, "Disabled"=w445) -> ("error out"=w449:errorcluster)  [unwired: 4 in, 7 out]
            n203 = call "Camera Update Slider Limits.vi"("Refnums"=w453, "Edit?"=w446, "error in (no error)"=w451, "Disabled"=w445) -> ("error out"=w448:errorcluster)  [unwired: 4 in, 7 out]
            n204 = call "Camera Update Slider Limits.vi"("Refnums"=w452, "Edit?"=w446, "error in (no error)"=w451, "Disabled"=w445) -> ("error out"=w447:errorcluster)  [unwired: 4 in, 7 out]
            n205 = Merge Errors(w449, w448, w447) -> (w450:errorcluster)
          }
          frame True {
            w479 = T8."Value" ("Edit?")
            w489 = T8."User Enablement" ("Edit?")
            w475 = u8 1
            w494 = 32771 items=["IS_GET_MASTER_GAIN"=32768, "IS_GET_RED_GAIN"=32769, "IS_GET_GREEN_GAIN"=32770, "IS_GET_BLUE_GAIN"=32771, "IS_GET_DEFAULT_MASTER"=32772, "IS_GET_DEFAULT_RED"=32773, "IS_GET_DEFAULT_GREEN"=32774, "IS_GET_DEFAULT_BLUE"=32775, "IS_SET_GAIN"=34816] ("Mode")
            w495 = 32770 items=["IS_GET_MASTER_GAIN"=32768, "IS_GET_RED_GAIN"=32769, "IS_GET_GREEN_GAIN"=32770, "IS_GET_BLUE_GAIN"=32771, "IS_GET_DEFAULT_MASTER"=32772, "IS_GET_DEFAULT_RED"=32773, "IS_GET_DEFAULT_GREEN"=32774, "IS_GET_DEFAULT_BLUE"=32775, "IS_SET_GAIN"=34816] ("Mode")
            w496 = 32769 items=["IS_GET_MASTER_GAIN"=32768, "IS_GET_RED_GAIN"=32769, "IS_GET_GREEN_GAIN"=32770, "IS_GET_BLUE_GAIN"=32771, "IS_GET_DEFAULT_MASTER"=32772, "IS_GET_DEFAULT_RED"=32773, "IS_GET_DEFAULT_GREEN"=32774, "IS_GET_DEFAULT_BLUE"=32775, "IS_SET_GAIN"=34816] ("Mode")
            w497 = 34820 items=["IS_SET_ENABLE_AUTO_GAIN"=34816, "IS_GET_ENABLE_AUTO_GAIN"=34817, "IS_SET_ENABLE_AUTO_SHUTTER"=34818, "IS_GET_ENABLE_AUTO_SHUTTER"=34819, "IS_SET_ENABLE_AUTO_WHITEBALANCE"=34820, "IS_GET_ENABLE_AUTO_WHITEBALANCE"=34821, "IS_SET_ENABLE_AUTO_FRAMERATE"=34822, "IS_GET_ENABLE_AUTO_FRAMERATE"=34823, "IS_SET_AUTO_REFERENCE"=32768, "IS_GET_AUTO_REFERENCE"=32769, "IS_SET_AUTO_GAIN_MAX"=32770, "IS_GET_AUTO_GAIN_MAX"=32771, "IS_SET_AUTO_SHUTTER_MAX"=32772, "IS_GET_AUTO_SHUTTER_MAX"=32773, "IS_SET_AUTO_SPEED"=32774, "IS_GET_AUTO_SPEED"=32775, "IS_SET_AUTO_WB_OFFSET"=32776, "IS_GET_AUTO_WB_OFFSET"=32777, "IS_SET_AUTO_WB_GAIN_RANGE"=32778, "IS_GET_AUTO_WB_GAIN_RANGE"=32779, "IS_SET_AUTO_WB_SPEED"=32780, "IS_GET_SUTO_WB_SPEED"=32781, "IS_SET_AUTO_WB_ONCE"=32782, "IS_GET_AUTO_WB_ONCE"=32783] ("Param")
            # "Auto Whitebalance"
            n206 = call <instrlib>:"SetAutoParameter.vi"("enable"=TRUE, "error in"=w501, "Param"=w497, "Camera Handle In"=w493) -> ("error out"=w500:errorcluster, "Camera Handle Out"=w504:u32)  [unwired: 1 in, 5 out]
            n207 = call <instrlib>:"SetHardwareGain.vi"("error in"=w500, "Mode"=w496, "Camera Handle In"=w504) -> ("error out"=w499:errorcluster, "Value"=w476:i32, "Camera Handle Out"=w503:u32)  [unwired: 4 in, 2 out]
            n208 = call <instrlib>:"SetHardwareGain.vi"("error in"=w499, "Mode"=w495, "Camera Handle In"=w503) -> ("error out"=w498:errorcluster, "Value"=w477:i32, "Camera Handle Out"=w502:u32)  [unwired: 4 in, 2 out]
            n209 = call <instrlib>:"SetHardwareGain.vi"("error in"=w498, "Mode"=w494, "Camera Handle In"=w502) -> ("error out"=w487:errorcluster, "Value"=w478:i32)  [unwired: 4 in, 3 out]
            n210 = Unbundle By Name(w486) -> ("Red Gain"=w490:refnum<vi>)
            n211 = Unbundle By Name(w486) -> ("Green Gain"=w491:refnum<vi>)
            n212 = Unbundle By Name(w486) -> ("Blue Gain"=w492:refnum<vi>)
            n213 = control-ref of="Red Gain"() -> (w471:refnum<vi>)
            n214 = control-ref of="Green Gain"() -> (w470:refnum<vi>)
            n215 = control-ref of="Blue Gain"() -> (w469:refnum<vi>)
            n216 = Build Array(w471, w490) -> (w474:refnum<vi>[])
            n217 = Build Array(w469, w492) -> (w472:refnum<vi>[])
            n218 = Build Array(w470, w491) -> (w473:refnum<vi>[])
            n219 = call "Camera Update Slider Limits.vi"("Refnums"=w474, "Edit?"=w489, "error in (no error)"=w487, "Disabled"=w475) -> ("error out"=w485:errorcluster)  [unwired: 4 in, 7 out]
            n220 = call "Camera Update Slider Limits.vi"("Refnums"=w473, "Edit?"=w489, "error in (no error)"=w487, "Disabled"=w475) -> ("error out"=w484:errorcluster)  [unwired: 4 in, 7 out]
            n221 = call "Camera Update Slider Limits.vi"("Refnums"=w472, "Edit?"=w489, "error in (no error)"=w487, "Disabled"=w475) -> ("error out"=w483:errorcluster)  [unwired: 4 in, 7 out]
            n222 = call "Camera Update Slider Limits.vi"("Refnums"=w474, "Edit?"=w479, "error in (no error)"=w485, "Value"=w476) -> ("error out"=w482:errorcluster)  [unwired: 4 in, 7 out]
            n223 = call "Camera Update Slider Limits.vi"("Refnums"=w473, "Edit?"=w479, "error in (no error)"=w484, "Value"=w477) -> ("error out"=w481:errorcluster)  [unwired: 4 in, 7 out]
            n224 = call "Camera Update Slider Limits.vi"("Refnums"=w472, "Edit?"=w479, "error in (no error)"=w483, "Value"=w478) -> ("error out"=w480:errorcluster)  [unwired: 4 in, 7 out]
            n225 = Merge Errors(w482, w481, w480) -> (w488:errorcluster)
          }
        }
        n226 = call <instrlib>:"SetAutoParameter.vi"("enable"=w390, "error in"=w409, "Param"=w405, "Camera Handle In"=w359) -> ("error out"=w408:errorcluster)  [unwired: 1 in, 6 out]
        n227 = case shown="False" w390 {
          tunnel: w408 -> [w426 w441]
          tunnel: [w417 w430] -> w355
          tunnel: w389 -> [w423 _]
          tunnel: w359 -> [w424 w439]
          tunnel: w352 -> [w416 w429]
          frame False {
            w425 = 34816 items=["IS_GET_MASTER_GAIN"=32768, "IS_GET_RED_GAIN"=32769, "IS_GET_GREEN_GAIN"=32770, "IS_GET_BLUE_GAIN"=32771, "IS_GET_DEFAULT_MASTER"=32772, "IS_GET_DEFAULT_RED"=32773, "IS_GET_DEFAULT_GREEN"=32774, "IS_GET_DEFAULT_BLUE"=32775, "IS_SET_GAIN"=34816] ("Mode")
            w427 = -1
            n228 = call <instrlib>:"SetHardwareGain.vi"("Blue"=w427, "Green"=w427, "Red"=w427, "error in"=w426, "Master Gain"=w423, "Mode"=w425, "Camera Handle In"=w424) -> ("error out"=w418:errorcluster)  [unwired: 4 out]
            n229 = Unbundle By Name(w416) -> ("Master Gain"=w422:refnum<vi>)
            n230 = control-ref of="Master Gain"() -> (w415:refnum<vi>)
            n231 = Build Array(w415, w422) -> (w421:refnum<vi>[])
            n232 = call "Camera Update Slider Limits.vi"("Refnums"=w421, "Edit?"=T8."User Enablement", "error in (no error)"=w418, "Disabled"=u8 0) -> ("error out"=w417:errorcluster)  [unwired: 4 in, 7 out]
          }
          frame True {
            w440 = 32768 items=["IS_GET_MASTER_GAIN"=32768, "IS_GET_RED_GAIN"=32769, "IS_GET_GREEN_GAIN"=32770, "IS_GET_BLUE_GAIN"=32771, "IS_GET_DEFAULT_MASTER"=32772, "IS_GET_DEFAULT_RED"=32773, "IS_GET_DEFAULT_GREEN"=32774, "IS_GET_DEFAULT_BLUE"=32775, "IS_SET_GAIN"=34816] ("Mode")
            # "On active AutoGain,\nSet Master Gain Slider Value"
            n233 = call <instrlib>:"SetHardwareGain.vi"("error in"=w441, "Mode"=w440, "Camera Handle In"=w439) -> ("error out"=w431:errorcluster, "Value"=w432:i32)  [unwired: 4 in, 3 out]
            n234 = Unbundle By Name(w429) -> ("Master Gain"=w437:refnum<vi>)
            n235 = control-ref of="Master Gain"() -> (w428:refnum<vi>)
            n236 = Build Array(w428, w437) -> (w438:refnum<vi>[])
            n237 = call "Camera Update Slider Limits.vi"("Refnums"=w438, "Edit?"=T8."User Enablement", "error in (no error)"=w431, "Disabled"=u8 1) -> ("error out"=w434:errorcluster)  [unwired: 4 in, 7 out]
            n238 = call "Camera Update Slider Limits.vi"("Refnums"=w438, "Edit?"=T8."Value", "error in (no error)"=w434, "Value"=w432) -> ("error out"=w430:errorcluster)  [unwired: 4 in, 7 out]
          }
        }
        n239 = Unbundle By Name(w353) -> ("Status"=w356:refnum<notifier>)
        n240 = Not A Number/Path/Refnum?(number/path/refnum=w356) -> (NaN/Path/Refnum?=w357:bool)
        n241 = case shown="True" w357 {
          tunnel: w355 -> [w413 w414]
          tunnel: [w412 w414] -> w354
          tunnel: w356 -> [w411 _]
          frame False {
            n242 = Send Notification(notification="Congifuration Updated", notifier=w411, error in (no error)=w413) -> (error out=w412:errorcluster)  [unwired: 1 out]
          }
          frame True {
          }
        }
      }
      frame "Acquire" {
        w516 = u32 0 items=["Horizontal", "Vertical", "Central", "1st Diagonal", "2nd Diagonal"] ("Type of Symmetry")
        n243 = call <instrlib>:"GetActImgMem.vi"("error in"=w535, "Camera Handle In"=w540) -> ("error out"=w532:errorcluster, "Image Memory Out"=w541:u8[])  [unwired: 8 out]
        n244 = Unbundle By Name(w539) -> ("Height"=w537:i32, "Width"=w538:i32, "Bits/Pixel"=w536:i32)
        n245 = call <instrlib>:"ArrayToVision.vi"("Bits/Pixel"=w536, "Height"=w537, "Width"=w538, "InArray"=w541) -> ("OutArray"=w518:u32[][])  [unwired: 1 in, 6 out]
        n246 = Bundle By Name(cluster=w539, "Image"=w518) -> (w534:T6)
        n247 = call "IMAQ ArrayToColorImage"("Image Pixels (U32)"=w518, "Image"=w533, "error in (no error)"=w532) -> ("Image Out"=w517:T3, "error out"=w522:errorcluster)  [unwired: 2 in]
        n248 = call "IMAQ Symmetry"("error in (no error)"=w522, "Type of Symmetry"=w516, "Image Dst"=w517, "Image Src"=w517) -> ("error out"=w514:errorcluster, "Image Dst Out"=w515:T3)  [unwired: 1 in]
        "Image" <- w515
        n249 = Unbundle By Name(w531) -> ("Image"=w529:refnum<vi>)
        n250 = Unbundle By Name(w523) -> ("Measurement"=w524:refnum<notifier>)
        n251 = Not A Number/Path/Refnum?(number/path/refnum=w529) -> (NaN/Path/Refnum?=w530:bool)
        n252 = Unbundle By Name(w523) -> ("Status"=w528:refnum<notifier>)
        n253 = case shown="False" w530 {
          tunnel: w514 -> [w555 w556]
          tunnel: [w554 w556] -> w519
          tunnel: w529 -> [w553 _]
          tunnel: w515 -> [w552 _]
          frame False {
            n254 = property class="ImageControl"(reference=w553, error in=w555, "Value"=w552) -> (error out=w554:errorcluster)  [unwired: 1 out]
          }
          frame True {
          }
        }
        n255 = Not A Number/Path/Refnum?(number/path/refnum=w524) -> (NaN/Path/Refnum?=w525:bool)
        n256 = case shown="False" w525 {
          tunnel: w514 -> [w550 w551]
          tunnel: [w549 w551] -> w526
          tunnel: w524 -> [w548 _]
          tunnel: w515 -> [w547 _]
          frame False {
            n257 = Send Notification(notification=w547, notifier=w548, error in (no error)=w550) -> (error out=w549:errorcluster)  [unwired: 1 out]
          }
          frame True {
          }
        }
        n258 = Not A Number/Path/Refnum?(number/path/refnum=w528) -> (NaN/Path/Refnum?=w527:bool)
        n259 = case shown="False" w527 {
          tunnel: w526 -> [w545 w546]
          tunnel: [w544 w546] -> w520
          tunnel: w528 -> [w543 _]
          frame False {
            n260 = Send Notification(notification="Image Acquired", notifier=w543, error in (no error)=w545) -> (error out=w544:errorcluster)  [unwired: 1 out]
          }
          frame True {
          }
        }
        n261 = Merge Errors(w520, w519) -> (w521:errorcluster)
      }
      frame "Disconnect" {
        n262 = call <instrlib>:"StopLiveVideo.vi"("Camera Handle In"=w558) -> ("error out"=w557:errorcluster)  [unwired: 2 in, 8 out]
        n263 = call <instrlib>:"ExitCamera.vi"("error in"=w557, "Camera Handle In"=w558) -> ("error out"=w573:errorcluster)  [unwired: 9 out]
        n264 = call "IMAQ Dispose"("Image"=w571) -> ("error out"=w570:errorcluster)  [unwired: 2 in, 3 out]
        n265 = Merge Errors(w570, w573, w574) -> (w563:errorcluster)
        n266 = Unbundle By Name(w566) -> ("Status"=w569:refnum<notifier>)
        n267 = Unbundle By Name(w561) -> ("Video Button"=w559:refnum<vi>)
        n268 = case shown="No Error" w563 {
          selector: w563 -> [w585 w590]
          tunnel: [w584 w589] -> w564
          tunnel: w561 -> [w581 w591]
          frame No Error {
            n269 = Unbundle By Name(w581) -> ("Instrument Status"=w582:refnum<vi>)
            n270 = control-ref of="Instrument Status"() -> (w580:refnum<vi>)
            n271 = Build Array(w582, w580) -> (w583:refnum<vi>[])
            n272 = call "Edit Status Indicator.vi"("error in (no error)"=w585, "State"=Instrument_Status_State."Disconnected", "Instrument Status Refnum"=w583) -> ("error out"=w584:errorcluster)  [unwired: 1 in, 7 out]
          }
          frame Error {
            n273 = Unbundle By Name(w591) -> ("Instrument Status"=w592:refnum<vi>)
            n274 = control-ref of="Instrument Status"() -> (w587:refnum<vi>)
            n275 = Build Array(w592, w587) -> (w593:refnum<vi>[])
            n276 = call "Edit Status Indicator.vi"("State"=Instrument_Status_State."Unknown", "Instrument Status Refnum"=w593) -> ("error out"=w588:errorcluster)  [unwired: 2 in, 7 out]
            n277 = Merge Errors(w588, w590) -> (w589:errorcluster)
          }
        }
        n278 = Not A Number/Path/Refnum?(number/path/refnum=w569) -> (NaN/Path/Refnum?=w568:bool)
        n279 = case shown="False" w568 {
          tunnel: w563 -> [w598 w599]
          tunnel: [w597 w599] -> w567
          tunnel: w569 -> [w596 _]
          frame False {
            n280 = Send Notification(notification="Disconnected", notifier=w596, error in (no error)=w598) -> (error out=w597:errorcluster)  [unwired: 1 out]
          }
          frame True {
          }
        }
        n281 = Not A Number/Path/Refnum?(number/path/refnum=w559) -> (NaN/Path/Refnum?=w560:bool)
        n282 = case shown="True" w560 {
          tunnel: [w577 w579] -> w562
          tunnel: w563 -> [w576 w579]
          tunnel: w559 -> [w575 _]
          frame False {
            n283 = property on="Property Node" class="Bool (strict)"(reference=w575, error in=w576, "Value"=FALSE ("Video")) -> (error out=w577:errorcluster)  [unwired: 1 out]
          }
          frame True {
          }
        }
        n284 = Merge Errors(w567, w562, w564) -> (w565:errorcluster)
      }
      frame "Stop Live" {
        n285 = disable-structure shown="Disabled" {
          disable-tunnel: [w613 _] -> w610
          disable-tunnel: w609 -> [w612 _]
          frame Disabled {
            n286 = call <instrlib>:"StopLiveVideo.vi"("Camera Handle In"=w612) -> ("error out"=w613:errorcluster)  [unwired: 2 in, 8 out]
          }
          frame Enabled {
          }
        }
        n287 = Merge Errors(w610, w611) -> (w602:errorcluster)
        n288 = case shown="No Error" w602 {
          selector: w602 -> [w619 w624]
          tunnel: [w618 w623] -> w600
          tunnel: w603 -> [w615 w625]
          frame No Error {
            n289 = Unbundle By Name(w615) -> ("Instrument Status"=w616:refnum<vi>)
            n290 = control-ref of="Instrument Status"() -> (w614:refnum<vi>)
            n291 = Build Array(w616, w614) -> (w617:refnum<vi>[])
            n292 = call "Edit Status Indicator.vi"("error in (no error)"=w619, "State"=Instrument_Status_State."Idle", "Instrument Status Refnum"=w617) -> ("error out"=w618:errorcluster)  [unwired: 1 in, 7 out]
          }
          frame Error {
            n293 = Unbundle By Name(w625) -> ("Instrument Status"=w626:refnum<vi>)
            n294 = control-ref of="Instrument Status"() -> (w621:refnum<vi>)
            n295 = Build Array(w626, w621) -> (w627:refnum<vi>[])
            n296 = call "Edit Status Indicator.vi"("State"=Instrument_Status_State."Unknown", "Instrument Status Refnum"=w627) -> ("error out"=w622:errorcluster)  [unwired: 2 in, 7 out]
            n297 = Merge Errors(w622, w624) -> (w623:errorcluster)
          }
        }
        n298 = Unbundle By Name(w604) -> ("Status"=w606:refnum<notifier>)
        n299 = Not A Number/Path/Refnum?(number/path/refnum=w606) -> (NaN/Path/Refnum?=w605:bool)
        n300 = case shown="False" w605 {
          tunnel: w602 -> [w632 w633]
          tunnel: [w631 w633] -> _
          tunnel: w606 -> [w630 _]
          frame False {
            n301 = Send Notification(notification="Live Stopped", notifier=w630, error in (no error)=w632) -> (error out=w631:errorcluster)  [unwired: 1 out]
          }
          frame True {
          }
        }
        n302 = Merge Errors(w602, w600) -> (w601:errorcluster)
      }
      frame "Update Refnums" {
        n303 = Unbundle By Name("Camera Notifiers") -> ("Status"=w637:refnum<notifier>)
        n304 = Not A Number/Path/Refnum?(number/path/refnum=w637) -> (NaN/Path/Refnum?=w636:bool)
        n305 = case shown="False" w636 {
          tunnel: w635 -> [w645 w646]
          tunnel: [w644 w646] -> _
          tunnel: w637 -> [w643 _]
          frame False {
            n306 = Send Notification(notification="Connected", notifier=w643, error in (no error)=w645) -> (error out=w644:errorcluster)  [unwired: 1 out]
          }
          frame True {
          }
        }
      }
    }
  }
  "Error Out" <- w6
  "Camera Handle" <- w2
  "Image" <- w3
